vi "AlliGator FLI Dataset Actions.vi"(0 "AlliGator Q Elements":T6[](array[typedef]), 1 "VI in":refnum<vi>, 2 "Script in":bool, 5 "AlliGator IV DVR in":refnum<data-value>, 7 "AlliGator Q Event in":T7=enum."GUI:Idle", 9 "Data":variant, 11 "error in (no error)":errorcluster, 12 "AlliGator Ctrl Refnums":T8) -> (3 "Script out":bool, 4 "Alligator Queue Elements":T6[](array[typedef]), 6 "AlliGator IV DVR out":refnum<data-value>, 10 "[Notebook Message]":T1[](array[typedef]) {"Message Style"."Font Size" min=6.0 step=1.0}, 15 "error out":errorcluster)   [LabVIEW 2021, in "AlliGator Action Engine.lvlib"]
doc: "Processes AlliGator FLI Dataset-related actions."
uses:
  AlliGator Action Engine.lvlib
  Internal Variables/AlliGator Internal Variables v2.ctl
  <vilib>/vision/Image Controls.llb/IMAQ Image.ctl
  Internal Variables/AlliGator Gate Image Set.ctl
  Files/AlliGator FLI Dataset Type.ctl
  Files/AlliGator Data Series Type.ctl
  Dual-Channel Datasets/AlliGator Dataset Channel.ctl
  Settings/AlliGator Gate Arithmetic.ctl
  Source Image/AlliGator Displayed Image.ctl
  Image/Named ROI Description.ctl
  Phasor Graph/AlliGator Decay Metadata v3.ctl
  Decay Analysis/Decay Preprocessing/AlliGator Decay Background Subtraction Info.ctl
  Decay Analysis/Decay Preprocessing/AlliGator Baseline Subtraction Method.ctl
  Graphs/XY Graph/XY Graph Plot Shift Parameters.ctl
  Graphs/XY Graph/XY Graph Plot Shift Method.ctl
  Decay Analysis/Decay Preprocessing/AlliGator Decay Extrapolation Parameters.ctl
  Phasor/Calibration Phasor (m, phi).ctl
  Phasor/Phasor Reference Series.ctl
  Phasor/Phasor Calibration Map v2.ctl
  Phasor/Phasor (g, s).ctl
  Phasor Graph/AlliGator Raw Phasor Plot Data v5.ctl
  Phasor/Phasor Standard Deviation Options.ctl
  Phasor Plot/AlliGator Phasor Multi-Harmonic Data.ctl
  Phasor/Phasor Harmonic Data.ctl
  Decay Fit Parameter Map/AlliGator Decay Fit Options & Parameters v3.ctl
  Fits/IRF(X)PSED/Decay Fit Options v3.ctl
  Fits/Decay Convolution/Decay Model.ctl
  Fits/Residual Type.ctl
  Fits/IRF(X)PSED/Fit Weights Type.ctl
  Fits/Non-linear Fitting Method v2.ctl
  Fits/Fit Calculation Method.ctl
  Fits/Non-linear Fitting Algorithm.ctl
  Decay Analysis/Decay Fit/AlliGator Decay Fit Parameter Constraints 2.ctl
  Fits/IRF(X)PSED/Decay Fit Parameters In List.ctl
  Fits/IRF(X)PSED/MLE Baseline Offset Type.ctl
  Decay Analysis/Decay Preprocessing/AlliGator Decay Preprocessing Parameters.ctl
  Fits/IRF(X)PSED/Decay Fit Parameters & Derived Quantities List v2.ctl
  Fits/IRF(X)PSED/Decay Fit Result Constraint.ctl
  Decay Fit Parameter Map/AlliGator Parameter Maps Data.ctl
  AlliGator Q Event.ctl
  GUI/AlliGator Ctrl Refnums.ctl
  GUI/AlliGator Other Ctrl Refnums.ctl
  GUI/AlliGator State Indicator.ctl
  GUI/AlliGator Main Window Tabs.ctl
  GUI/AlliGator Phasor Plot Ctrl Refnums.ctl
  GUI/AlliGator Phasor Graph Ctrl Refnums.ctl
  Phasor/Phasor Calibration Type.ctl
  GUI/AlliGator Dataset Ctrl Refnums.ctl
  GUI/AlliGator Registered Events Ctrl Refnums.ctl
  GUI/AlliGator Image Histogram Control Refnums.ctl
  Histograms/Linear Histogram Options.ctl
  Histograms/Histogram Bin Option.ctl
  Histograms/Histogram Bin Position.ctl
  Decay Fit Parameter Map/AlliGator Decay Fit Map Control Refnums.ctl
  Parameter Map/AlliGator Parameter Map Control Refnums.ctl
  AlliGator Q Element.ctl
  Notebook/Notebook Message Object.ctl
  Rich Text Box/Text Formatting.ctl
  Rich Text Box/Text Colors.ctl
  Rich Text Box/Text Style.ctl
  Rich Text Box/Text Alignment.ctl
  AlliGator State Indicators List.ctl
  Alligator Elements Order in Action Stack.ctl
  Rich Text Box/Text Format List.ctl
  Graphs/Plot Point Style.ctl
  Graphs/LabVIEW Plot Interpolation.ctl
  Files/Load-Save File Info.ctl
  Dual-Channel Datasets/AlliGator Channel Arithmetic Action Parameters.ctl
  Scripts/AlliGator Multi-ROIs Dialog Type.ctl
  Image/Image Control ROI Description.ctl
  AlliGator Add Action Array to Stack.vi
  Variant/Variant to Data/Variant to Boolean.vi
  Graphs/XY Graph/XY Graph Add Single Plot with Name.vi
  Variant/Variant to Data/Variant to String.vi
  Image/Image.lvlib
  ROIs/AlliGator ROIs.lvlib
  Variant/Variant.lvlib
  Variant/Variant to Data/Variant to Data.lvlib
  GUI/GUI.lvlib
  Settings/AlliGator Settings.lvlib
  Dual-Channel Datasets/AlliGator Dual-Channel Datasets.lvlib
  Python Plugins API/AlliGator Python Plugins.lvlib
  Sound/Sound.lvlib
  Source Image/AlliGator Source Image.lvlib
  Scripts/AlliGator Scripts.lvlib
  Decay Analysis/IRF/AlliGator IRF.lvlib
  GUI/AlliGator GUI.lvlib
  Decay Analysis/Decay Fit/AlliGator Decay Fit.lvlib
  Decay Statistics/AlliGator Decay Statistics.lvlib
  Internal Variables/AlliGator Internal Variables.lvlib
  Decay Analysis/Decay Processing/AlliGator Decay Processing.lvlib
  Error/Error.lvlib
  Decay Fit Parameter Map/AlliGator Decay Fit Parameter Map.lvlib
  Phasor Graph/AlliGator Phasor Graph.lvlib
  Graphs/Graphs.lvlib
  Graphs/XY Graph/XY Graph Add-Ons.lvlib
  Files/Files.lvlib
  Notebook/Notebook.lvlib
  Phasor/Phasor.lvlib
  Decay Analysis/Decay Preprocessing/AlliGator Decay Preprocessing.lvlib
  Files/AlliGator Files.lvlib
  Phasor Plot/AlliGator Phasor Plot.lvlib
  Fits/Fits.lvlib
  Rich Text Box/Rich Text Box.lvlib
  Histograms/Histogram Window.lvlib
  Parameter Map/AlliGator Parameter Map.lvlib
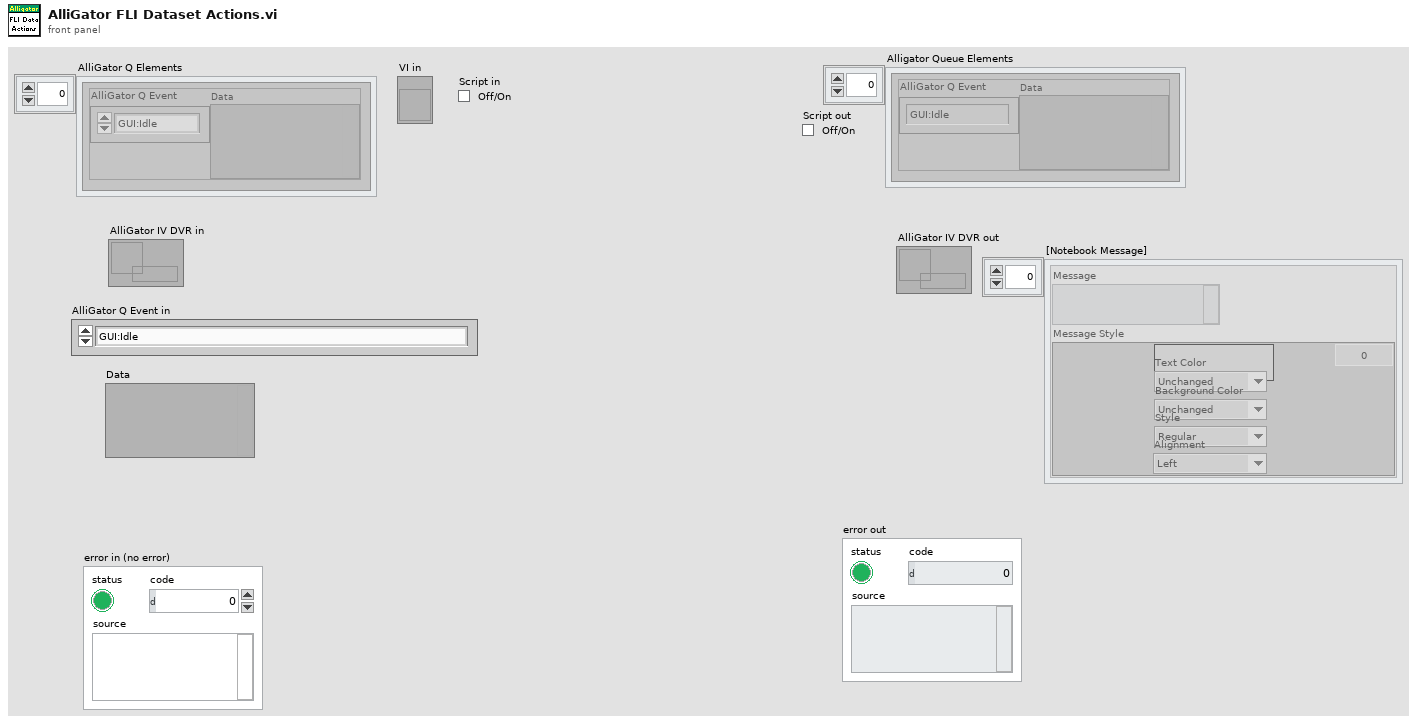
[diagram p1: front panel]
types:
  T1 = typedef "Notebook.lvlib/Notebook Message Object.ctl" = cluster{"Message":string, "Message Style":T2}
  T2 = typedef "Rich Text Box.lvlib/Text Formatting.ctl" = cluster{"Font":string, "Text Color":T3, "Background Color":T3, "Style":T4, "Font Size":dbl, "Alignment":T5}
  T3 = typedef "Rich Text Box.lvlib/Text Colors.ctl" = enum16{"Unchanged", "Black", "Blue", "Cyan", "Maroon", "Gray", "Violet", "Green", "Light Green", "Orange", "Yellow", "Magenta", "Red", "White"}
  T4 = typedef "Rich Text Box.lvlib/Text Style.ctl" = enum16{"Regular", "Bold", "Italic", "Underline", "Strikeout"}
  T5 = typedef "Rich Text Box.lvlib/Text Alignment.ctl" = enum16{"Left", "Right", "Center"}
  T6 = typedef "AlliGator Action Engine.lvlib/AlliGator Q Element.ctl" = cluster{"AlliGator Q Event":T7, "Data":variant}
  T7 = typedef "AlliGator Action Engine.lvlib/AlliGator Q Event.ctl" = enum16{"---- Files ----", "Files:Set Batch Export Files To Save", "Files:Set Dataset Loading & Pre-processing Options", "Files:Check #Frames in Dataset", "Files:Increment Frame Index", "Files:Open Mask Image", "Files:Open White Light Image", "Files:Open Single Dataset", "Files:New Folder of Folders Selected", "Files:Load File (all Types)_Scriptable", "Files:Move Flattened Series to Folders Series", "Files:Select Folder", "Files:Load FLI Dataset", "Files:Load Swiss SPAD 1 Dataset", "Files:Load Swiss SPAD 2 Dataset", "Files:Load .sdt FLI Dataset", "Files:Load .ptu FLI Dataset", "Files:Load .bin FLI Dataset", "Files:Load Single Gate Image Folder", "Files:Load I/m/phi Dataset (deprecated)", "Files:Load Single Image", "Files:Subtract Background File", "Files:Export FLI Dataset", "Files:Load HDF5 FLI Dataset", "Files:Set Destination File Path", "Files:Save Mask Image", "Files:Batch Conversion", "Files:New Folder Selected", "Files:Close FLI Dataset", "Files:Close FLI Dataset Series", "Files:Close White Light Image", "Files:Close Mask Image", "---- FLI Dataset ----", "FLI Dataset:Channel Arithmetic", "FLI Dataset:Export Average Lifetime Map as ASCII", "FLI Dataset:Export User-Defined Quantity Map as ASCII", "FLI Dataset:Python Function FLI Dataset Event", "FLI Dataset:ROI Analysis", "FLI Dataset:Tilted Logistic Square Gated IRF Characteristics Map", "FLI Dataset:Logistic Square Gated IRF Characteristics Map", "FLI Dataset:Square Gated IRF Characteristics Map", "FLI Dataset:Multi-ROI Single-Pixel Phasor Analysis", "FLI Dataset:Multi-ROI Single-Pixel NLSF Analysis", "FLI Dataset:All ROIs IRF Extraction", "FLI Dataset:All ROIs Decay Fit Non-Interactive (Fast + Individual IRF)", "FLI Dataset:All ROIs Phasor Analysis", "FLI Dataset:All ROIs Decay Fit", "FLI Dataset:Fluorescence Decay Statistics", "FLI Dataset:Update Decay Statistics Graph", "FLI Dataset:Get Decay from ROI", "FLI Dataset:All ROIs Average Lifetimes", "FLI Dataset:Save/Load Local IRFs", "FLI Dataset:Clear Local IRFs", "FLI Dataset:Phasor Calibration Maps (# Gates Series) Script", "FLI Dataset:Calibrated Phasor Map Series", "---- FLI Dataset Series ----", "FLI Dataset Series:Sum All Datasets in Series", "FLI Dataset Series:Add Dataset to Accumulated Dataset", "FLI Dataset Series:Display Accumulated Dataset", "FLI Dataset Series:Clear Dataset Series Sum", "FLI Dataset Series:Time-Series Analysis (NLSF)", "FLI Dataset Series:Time-Series Analysis (Phasor)", "---- Image ----", "Image:Update Image Profile Plots", "Image:Image Histogram Cursor Move", "Image:Image Histogram", "Image:Image Contrast", "Image:Set Image Histogram Cursor Move Flag", "Image:Clear Image Overlay", "Image:Use ROI as Search Area", "Image:Set ROI Diameter", "Image:Save Image Data as TIFF", "Image:Save Displayed Image with Overlay", "Image:Save Image Overlay Only", "Image:Save Image as Hot Pixel Mask", "Image:Change Source Image Color Palette", "Image:Copy Image to Clipboard", "Image:Source Image ROI Selection", "Image:Delete All ROIs", "Image:Delete All Unselected ROIs", "Image:Delete ROI", "Image:Merge All ROIs", "Image:Store ROI", "Image:Source Image ROI Storage", "Image:Export ROI Description to Notebook", "Image:Save ROI", "Image:Load ROI", "Image:Paste ROI Definition", "Image:Clear ROI", "Image:Identify ROIs in Mask Image", "Image:Create Complementary ROI", "Image:Create Contour ROI", "Image:Create ROI(s) from Pixels with Peak above Min_Scriptable", "Image:Create ROI(s) from Pixels with Intensity above Min_Scriptable", "Image:Compute ROI Statistics", "Image:Delete ROI(s) based on ROI Characteristics", "Image:Create ROI Grid", "Image:ROI to Individual Pixel ROIs", "Image:Python Function Source Image Event", "Image:Show Phasor Calibration Map ROI Centers", "Image:Convert ROI to Mask Image", "Image:Mouse Move", "Image:Mouse Up", "Image:Set Source Image Mouse Move Flag", "Image:Add Scale Bar Overlay", "Image:Delete Existing ROIs Option", "Image:Overlay ROI Median", "Image:Check Current ROI", "Image:Update True Pixel Value", "---- Decay ----", "Decay:Clear IRF/Reference Plot", "Decay:Add Decay to Graph", "Decay:Smoothen Plot", "Decay:Smoothen Plot Tail", "Decay:Average Selected Plots", "Decay:Extract IRF", "Decay:Optimal IRF Extraction", "Decay:Threshold IRF", "Decay:Fit to Model IRF", "Decay:Fit IRF to Square Gate", "Decay:Fit IRF to Logistic Square Gate", "Decay:Fit IRF to Tilted Logistic Square Gate", "Decay:Create Bounding Cursors Set", "Decay:Export Bounding Cursors Definition to Notebook", "Decay:Denoise Plot", "Decay:Compute Cumulative Function", "Decay:Use as Reference Decay", "Decay:Show Reference Decay/IRF", "Decay:Extrapolate Decay", "Decay:Create Head & Tail Bounding Cursors", "Decay:Store Cursor-defined Head & Tail Fractions", "Decay:Rebin Plot", "Decay:1-Normalize Decay", "Decay:[0-1]-Normalize Plot", "Decay:Straighten Decay", "Decay:Shift Decay", "Decay:Fold Decay", "Decay:Fit Decay", "Decay:Global Fit of Selected Decays", "Decay:Post Global Fit Script", "Decay:Add Global Fit Parameters to Graph", "Decay:Add Decay Parameter(s) to Plot (Graph)", "Decay:Export Decay to Phasor Graph", "Decay:Compute Average Lifetime", "Decay:Plot Convolution", "Decay:Graph Tip Strip Update", "---- Decay Statistics ----", "Decay Statistics:Tip Strip Update", "---- Intensity Time Trace ----", "Intensity Time Trace:Use File Timestamp", "Intensity Time Trace:Load Intensity Corrections File", "Intensity Time Trace:Clear Intensity Corrections File", "Intensity Time Trace:Tip Strip Update", "---- Phasor Plot ----", "Phasor Plot:Build Phasor Plot", "Phasor Plot:Change Phasor Plot Color Palette", "Phasor Plot:Adjust Phasor Plot Display Range", "Phasor Plot:Highlight Image ROI in Phasor Plot", "Phasor Plot:Save Phasor Plot Image with Overlay", "Phasor Plot:Export Complex Phasor Map", "Phasor Plot:Export Phasor Ratio Map", "Phasor Plot:Export Average Lifetime Map", "Phasor Plot:Compute Phase Lifetime Histogram", "Phasor Plot:Compute Phasor Ratio Histogram", "Phasor Plot:Compute Phase Lifetime vs Intensity Scatter Plot", "Phasor Plot:Weber 2-Component Decomposition", "Phasor Plot:Update Phasor Color Map Vertices", "Phasor Plot:Clear Phasor Overlay", "Phasor Plot:Use Segment Extremities as References", "Phasor Plot:Use UC/Segment Intersections as References", "Phasor Plot:Use UC/Principal Axis Intersections as References", "Phasor Plot:Use UC/Linear Fit Intersections as References", "Phasor Plot:Update Phasor Plot Reference", "Phasor Plot:Show Local Phasor Info in Phasor Plot", "Phasor Plot:Update Phasor Plot State", "Phasor Plot:Phasor Plot ROI Storage", "Phasor Plot:Phasor Plot ROI Selection", "Phasor Plot:Python Function Phasor Plot Event", "Phasor Plot:Overlay Phasor ROI, Ratio or Map in Source Image", "Phasor Plot:Compute Decay of Selected Phasors", "Phasor Plot:Phasor at Image Pixel", "Phasor Plot:Mouse Move", "Phasor Plot:Mouse Up", "Phasor Plot:Display Range Mouse Move", "Phasor Plot:Set Mouse Move Flag", "Phasor Plot:Update True Phasor Plot Value", "---- Phasor Graph ----", "Phasor Graph:Get Phasor Value", "Phasor Graph:Create New Phasor Plot Dialog", "Phasor Graph:Update Last Phasor Value", "Phasor Graph:Update Phasor (m, phi)", "Phasor Graph:Remove Single Phasor from Plot", "Phasor Graph:Add Single Phasor to Plot", "Phasor Graph:Remove Phasor Plot", "Phasor Graph:Remove Selected Phasor Plots", "Phasor Graph:Clear Phasor Data", "Phasor Graph:Clear Phasor Graph", "Phasor Graph:Cursor Move", "Phasor Graph:Draw Cursor Connecting Line", "Phasor Graph:Clear Cursor Connecting Line", "Phasor Graph:Find UC Intersection", "Phasor Graph:Use UC/Cursor-Defined Line Intersections", "Phasor Graph:Use Selected Plots Fitted Line/UC Intersections", "Phasor Graph:Use Selected Plots Principal Axis/UC Intersections", "Phasor Graph:Show Single Phasor", "Phasor Graph:Save Single Phasor Plot", "Phasor Graph:Save All Phasor Plots", "Phasor Graph:Load Phasor Plot(s)", "Phasor Graph:Phasor Multiplication", "Phasor Graph:Compute Average Phasor", "Phasor Graph:Compute Multiple Average Phasors (Selected Plots)", "Phasor Graph:Export Single Phasor Plot Phase Lifetimes", "Phasor Graph:Parameter 2 vs Parameter 1 Scatter Plot", "Phasor Graph:Use Cursor n Location", "Phasor Graph:Set Reference n to Current Phase Lifetime Value", "Phasor Graph:Set Reference n to Lifetime Value", "Phasor Graph:Set Cursor n Location", "Phasor Graph:Save Phasor Graph Image", "Phasor Graph:Update SEPL Plot", "Phasor Graph:Export Single Phasor Plot Data", "Phasor Graph:Export Selected Phasor Plots Data", "Phasor Graph:Python Function Phasor Graph Event", "Phasor Graph:Tip Strip Update", "---- Calibration ----", "Calibration:Set Calibration Type", "Calibration:Load/Save Phasor Calibration", "Calibration:Load/Save Phasor Calibration Series", "Calibration:Load/Save Phasor Calibration Map", "Calibration:Use as Calibration", "Calibration:Compute Optimal Calibration from Phasor References", "Calibration:Clear Phasor Calibration", "Calibration:Single Phasor Calibration Information", "Calibration:Use as Calibration Series", "Calibration:Use as Calibration Map", "Calibration:Clear Calibration Series", "Calibration:Phasor Calibration Series Information", "Calibration:Clear Calibration Map", "Calibration:Phasor Calibration Map Information", "Calibration:Apply Phasor Calibration", "Calibration:Update Single Plot Calibration", "Calibration:Update Multiple Plots Calibration", "Calibration:Clear Single Plot Calibration", "Calibration:Clear All Plots Calibrations", "Calibration:Clear Plot(s) Calibration(s)?", "---- Phasor Ratio ----", "Phasor Ratio:Clear Reference n", "Phasor Ratio:Toggle Selected Plot(s)  Lock to Reference 1", "Phasor Ratio:Use as Reference n", "Phasor Ratio:Send Reference n to Notebook", "Phasor Ratio:Toggle Selected Plot(s)  Lock to Reference 2", "Phasor Ratio:Compute Phasor Ratio at Mouse Location", "Phasor Ratio:Compute Phasor Plot's Average Phasor Ratio", "Phasor Ratio:Compute Time-Series Phasor Ratios", "Phasor Ratio:Fit Line to Phasor Ratio Plot", "Phasor Ratio:Save References", "Phasor Ratio:Load References", "Phasor Ratio:Update Phasor Reference 1", "Phasor Ratio:Update Phasor Reference 2", "Phasor Ratio:Move Cursor n to Reference n", "Phasor Ratio:Use as Phasor Reference 1 Lifetime", "Phasor Ratio:Use as Phasor Reference 2 Lifetime", "Phasor Ratio:Export Phasor Ratio Map as ASCII", "Phasor Ratio:Tip Strip Update", "---- Lifetime & Other Parameters Graph ----", "Lifetime:Compute Sliced Mean, SDV and CV Plots", "Lifetime:Plot Decay Shifts", "Lifetime:Plot Histogram", "---- Decay Fit Parameter Map ----", "Decay Fit Parameter Map:Export ROI NLSF Data as ASCII", "Decay Fit Parameter Map:Set Decay Fit Parameter Map Selection", "Decay Fit Parameter Map:Build Decay Fit Parameter Map", "Decay Fit Parameter Map:Change Decay Fit Parameter Map Color Palette", "Decay Fit Parameter Map:Export Decay Fit Parameter Map Data as ASCII", "Decay Fit Parameter Map:Export All Decay Fit Parameter Maps Data as ASCII", "Decay Fit Parameter Map:Selected Parameter Scatterplot", "Decay Fit Parameter Map:Parameter 2 vs Parameter 1 Scatterplot", "Decay Fit Parameter Map:Save Decay Fit Parameter Map Image", "Decay Fit Parameter Map:Save-Load IRFs & Fit Data", "Decay Fit Parameter Map:Update Local Decay Plots", "Decay Fit Parameter Map:Python Function Decay Fit Parameters Map Event", "Decay Fit Parameter Map:Overlay Decay Fit Parameter Map in Source Image", "Decay Fit Parameter Map:Selected Parameter vs Intensity Scatterplot", "Decay Fit Parameter Map:Mouse Up", "Decay Fit Parameter Map:Mouse Move", "Decay Fit Parameter Map:Display Range Mouse Move", "Decay Fit Parameter Map:Change Map Resolution", "Decay Fit Parameter Map:Variance Significance Maps", "Decay Fit Parameter Map:Fit Result Constraints Window", "---- Parameter Map ----", "Parameter Map:Export ROI Parameters Data as ASCII", "Parameter Map:Delete Parameter Map Set", "Parameter Map:Update Parameter List", "Parameter Map:Build Parameter Map", "Parameter Map:Change Parameter Map Color Palette", "Parameter Map:Export Parameter Map Data as ASCII", "Parameter Map:Export All Parameter Maps Data as ASCII", "Parameter Map:Selected Parameter Scatterplot", "Parameter Map:Parameter 2 vs Parameter 1 Scatterplot", "Parameter Map:Selected Parameter vs Intensity Scatterplot", "Parameter Map:Save Parameter Map Image", "Parameter Map:Save-Load IRFs & Parameter Maps (TODO)", "Parameter Map:Set Parameter Map Selection", "Parameter Map:Python Function Parameter Map Event", "Parameter Map:Overlay Parameter Map in Source Image", "Parameter Map:Update Local Decay Plots", "Parameter Map:Mouse Up", "Parameter Map:Mouse Move", "Parameter Map:Display Range Mouse Move", "---- Generic Graph ----", "Generic Graph:Generic XY Graph Event", "Generic Graph:Python Function XY Graph Event", "Generic Graph:New Plot", "Generic Graph:Save Plot", "Generic Graph:XY Plot Histogram", "Generic Graph:Set XY Graph Plot Name", "Generic Graph:Set Last Cursor Style", "Generic Graph:Tip Strip Update", "---- GUI ----", "GUI:Start Script", "GUI:Type of Displayed Image Changed", "GUI:Gate Image Slide Changed", "GUI:Show Busy Icon", "GUI:Show Busy Icon & Abort Button", "GUI:Hide Busy Icon", "GUI:Hide Busy Icon & Abort Button", "GUI:Abort", "GUI:End Script", "GUI:Start Timing", "GUI:End Timing", "GUI:Set State Indicator", "GUI:Send Parameters JSON Strings to Clipboard", "GUI:Set Gate Step", "GUI:Idle", "GUI:Initialization", "GUI:Quit", "GUI:Increment Dataset Index", "GUI:Set Dataset Index to -1", "GUI:Time Series Slider Moved", "GUI:Time Series Slider Changed", "GUI:Toggle Playback or Loop", "GUI:Playback Script", "GUI:Set Phasor Frequency", "GUI:Open Window", "GUI:Start Test Script", "GUI:End Test Script", "GUI:Set Verbose Mode", "GUI:Set Verbose Settings Mode", "DEBUG"}
  T8 = typedef "AlliGator GUI.lvlib/AlliGator Ctrl Refnums.ctl" = cluster{"Other AlliGator Ctrl Refnums":T9, "Phasor Plot Ctrl Refnums":T10, "Phasor Graph Ctrl Refnums":T11, "Dataset Control Refnums":T12, "Registered Events Ctrl Refnums":T13, "Image Histogram Ctrl Refnums":T14, "Decay Fit Map Ctrl Refnums":T15, "Parameter Map Ctrl Refnums":T16}
  T9 = typedef "AlliGator GUI.lvlib/AlliGator Other Ctrl Refnums.ctl" = cluster{"State Indicators":refnum<vi>, " Progress Bar":refnum<vi>, "Decay Graph Active":refnum<vi>, "Decay Statistics Bin":refnum<vi>, "Time Step":refnum<vi>, "Use File Timestamp":refnum<vi>, "Tab Control":refnum<vi>, "CPU":refnum<vi>, "Abort Fit":refnum<vi>, "Dataset File/Folder Path":refnum<vi>, "Abort ROI Creation":refnum<vi>, "Event LED":refnum<vi>, "Dataset File/Folder Path 2":refnum<vi>, "Dataset File/Folder Path 3":refnum<vi>, "Dataset File/Folder Path 4":refnum<vi>, "Dataset File/Folder Path 5":refnum<vi>, "Dataset File/Folder Path 6":refnum<vi>, "Dataset File/Folder Path 7":refnum<vi>, "Dataset File/Folder Path 8":refnum<vi>, "Dataset File/Folder Path 9":refnum<vi>, "Dataset File/Folder Path 10":refnum<vi>, "Dataset File/Folder Path 11":refnum<vi>}
  T10 = typedef "AlliGator GUI.lvlib/AlliGator Phasor Plot Ctrl Refnums.ctl" = cluster{"Phasor Ratio":refnum<vi>, "Modulus Lifetime":refnum<vi>, "Phasor at cursor (m, phi)":refnum<vi>, "Phase Lifetime":refnum<vi>, "Phasor at cursor (g, s)":refnum<vi>, "Phasor Plor Average Lifetime":refnum<vi>, "Phasor Plot Active":refnum<vi>, "Save Phasor Plot":refnum<vi>, "Image Overlay Color":refnum<vi>, "Phasor Plot Color Scale":refnum<vi>, "Reference 1 Button":refnum<vi>, "Reference 2 Button":refnum<vi>, "True Phasor Plot Value":refnum<vi>}
  T11 = typedef "AlliGator GUI.lvlib/AlliGator Phasor Graph Ctrl Refnums.ctl" = cluster{"Phasor Ratio":refnum<vi>, "Modulus Lifetime":refnum<vi>, "Phasor at cursor (m, phi)":refnum<vi>, "Phase Lifetime":refnum<vi>, "Phasor at cursor (g, s)":refnum<vi>, "Phasor Graph Average Lifetime":refnum<vi>, "Phasor Graph Active":refnum<vi>, "Save Phasor Graph":refnum<vi>, "Phasor Frame Slide":refnum<vi>, "Single Step Phasor":refnum<vi>, "Calibration Type":refnum<vi>, "Show Line":refnum<vi>, "Phase Lifetime 1":refnum<vi>, "Phase Lifetime 2":refnum<vi>, "Phasor Graph Frequency":refnum<vi>, "Phasor Reference 1 Control":refnum<vi>, "Phasor Reference 2 Control":refnum<vi>, "Calibration Lifetime":refnum<vi>, "Phase Lifetime SDV":refnum<vi>, "Average Lifetime SDV":refnum<vi>, "Phasor Ratio SDV":refnum<vi>, "Modulus Lifetime SDV":refnum<vi>}
  T12 = typedef "AlliGator GUI.lvlib/AlliGator Dataset Ctrl Refnums.ctl" = cluster{"Current Data":refnum<vi>, "Gate Image Slide":refnum<vi>, "Time Point Slide":refnum<vi>, "Current Time Stamp":refnum<vi>, "Save Image":refnum<vi>, "Displayed Image":refnum<vi>, "Overlay Mode":refnum<vi>, "Phasor Overlay Color":refnum<vi>, "Image Color Scale":refnum<vi>, "Use ROI as Search Area":refnum<vi>, "Source Image ROI Color":refnum<vi>, "True Pixel Value":refnum<vi>}
  T13 = typedef "AlliGator GUI.lvlib/AlliGator Registered Events Ctrl Refnums.ctl" = cluster{"Time Point Slider":refnum<vi>, "Phasor Plot Display Range":refnum<vi>, "Decay Graph":refnum<vi>, "Decay Statistics Graph":refnum<vi>, "Intensity Time Trace":refnum<vi>, "Phasor Graph":refnum<vi>, "Phasor Ratio Graph":refnum<vi>, "Lifetime Graph":refnum<vi>, "Phasor Plot Display":refnum<vi>, "Source Image Display":refnum<vi>, "Decay Fit Parameter Map Display Range":refnum<vi>, "Decay Fit Parameter Map Display":refnum<vi>, "Parameter Map Display Range":refnum<vi>, "Parameter Map Display":refnum<vi>, "Phasor Plot Display Range":refnum<vi>}
  T14 = typedef "AlliGator GUI.lvlib/AlliGator Image Histogram Control Refnums.ctl" = cluster{"Image Histogram":refnum<vi>, "Image Histogram Options":refnum<vi>, "Image Histogram Active":refnum<vi>, "Image Histogram Upper Percentile":refnum<vi>, "Image Histogram Lower Percentile":refnum<vi>, "Auto-Adjust Contrast":refnum<vi>}
  T15 = typedef "AlliGator Decay Fit Parameter Map.lvlib/AlliGator Decay Fit Map Control Refnums.ctl" = cluster{"Decay Fit Parameter Map Color Scale":refnum<vi>, "Decay Fit Parameter":refnum<vi>, "Max Parameter":refnum<vi>, "Min Parameter":refnum<vi>, "Decay Fit Parameter Map Display":refnum<vi>, "Decay Fit Parameter Map Display Range":refnum<vi>, "Decay Parameter Map X":refnum<vi>, "Decay Parameter Map Y":refnum<vi>, "Decay Parameter Map Value":refnum<vi>}
  T16 = typedef "AlliGator Parameter Map.lvlib/AlliGator Parameter Map Control Refnums.ctl" = cluster{"Parameter Map Color Scale":refnum<vi>, "Map Parameter":refnum<vi>, "Max Parameter":refnum<vi>, "Min Parameter":refnum<vi>, "Parameter Map Display":refnum<vi>, "Parameter Map Display Range":refnum<vi>, "Parameter Map Set":refnum<vi>, "Parameter Map X":refnum<vi>, "Parameter Map Y":refnum<vi>, "Parameter Map Value":refnum<vi>}
  T17 = typedef "Notebook.lvlib/Text Format List.ctl" = enum16{"Message", "Result", "Error", "Setting", "Verbose", "Warning"}
  T18 = typedef "AlliGator Action Engine.lvlib/Alligator Elements Order in Action Stack.ctl" = enum16{"Enqueue 2 AFTER 1", "Enqueue 2 BEFORE 1"}
  T19 = typedef "AlliGator Action Engine.lvlib/AlliGator State Indicators List.ctl" = enum16{"Phasor Calibration Defined", "Phasor Calibration Series Defined", "Phasor Calibration Map Defined", "Phasor Reference 1 Defined", "Phasor Reference 2 Defined", "Lifetime Reference 1 Defined", "Lifetime Reference 2 Defined", "Phasor Calibration Used", "Phasor Calibration Series Used", "Phasor Calibration Map Used", "Dataset Update Needed", "Phasor Plot Update Needed", "Reference/IRF Defined", "Individual IRFs Defined"}
  T20 = typedef "Graphs.lvlib/LabVIEW Plot Interpolation.ctl" = enum16{"Point (.)", "Stepwise Right (--.)", "Line + Point (\\. /)", "Stepwise Left (.--)", "Stepwise Centered (-.-)", "Stepwise Vertical (|.|)", "Line (-)", "Use Previous Plot's Style"}
  T21 = typedef "Graphs.lvlib/Plot Point Style.ctl" = enum16{"not defined", "None", "Empty Circle", "Filled Circle", "Thick Circle", "Dotted Circle", "Empty Square", "Filled Square", "Thick Square", "Dotted Square", "Small Filled Square", "Dot", "Cross", "Tiny Cross", "Large X", "Small x", "Diamond", "Small Empty Square"}
  T22 = typedef "Files.lvlib/Load-Save File Info.ctl" = cluster{"Load/Save":bool, "File Path":path}
  T23 = typedef "AlliGator Dual-Channel Datasets.lvlib/AlliGator Channel Arithmetic Action Parameters.ctl" = cluster{"Channel Name":u16, "Channel Arithmetic":T24}
  T24 = typedef "AlliGator Settings.lvlib/AlliGator Gate Arithmetic.ctl" = enum16{"None", "INT-G2", "G2/INT*<INT>", "(1 - G2/INT)*<INT>"}
  T25 = typedef "ROI Descriptor" = cluster{"Global Rectangle":i32[], "Contours":cluster{"ID":enum32{"External", "Internal"}, "Type":u32, "Coordinates":i32[]}[]}
  T26 = typedef "AlliGator Scripts.lvlib/AlliGator Multi-ROIs Dialog Type.ctl" = enum16{"Multi-ROIs Single-Pixel Phasor Analysis", "Multi-ROIs Single-Pixel NLSF Analysis", "Export ROI Fit Parameters as ASCII"}
  T27 = typedef "Image.lvlib/Image Control ROI Description.ctl" = cluster{"Image Control Label":string, "ROI Descriptor":T25}
  T28 = typedef "AlliGator GUI.lvlib/AlliGator State Indicator.ctl" = cluster{"Phasor Calibration Defined":bool, "Phasor Calibration Series Defined":bool, "Phasor Calibration Map Defined":bool, "Phasor Ratio Reference 1 Defined":bool, "Phasor Ratio Reference 2 Defined":bool, "Phasor Ratio Lifetime Reference 1 Defined ":bool, "Phasor Ratio Lifetime Reference 2 Defined":bool, "Phasor Calibration Used":bool, "Phasor Calibration Series Used":bool, "Phasor Calibration Map Used":bool, "Dataset Update Needed":bool, "Phasor Plot Update Needed":bool, "Reference/IRF Defined":bool, "Individual IRFs Defined":bool}
  T29 = typedef "IMAQ Image.ctl" = refnum<image>
  T30 = typedef "AlliGator Scripts.lvlib/AlliGator Data Load & Process Options.ctl" = cluster{"Data Information":T31, "Source Image Settings":T35, "Decay Preprocessing Options & Parameters":T42, "Clear Phasor Graph":bool}
  T31 = typedef "AlliGator Scripts.lvlib/AlliGator Data Information.ctl" = cluster{"Gates to Skip":T32, "# Gates":u32, "Gate Step":u32, "Gate Duration":dbl[unit], "Gate Separation":dbl[unit], "Pile-up Correction":bool, "Pixel Well Capacity":u32, "Define Gates to":T33, "Gates to Keep":T34, "Laser Period":dbl[unit], "SYNC Period":dbl[unit], "Channel Name":u16, "Channel Arithmetic":T24, "Background File Subtraction":bool, "Background Scaling Factor":dbl, "Background File":path, "Background Pile-up Correction":bool, "Background Pixel Well Capacity":u32, "Dataset Scaling Factor":dbl}
  T32 = typedef "AlliGator Settings.lvlib/AlliGator Background Subtraction Parameters.ctl" = cluster{"Start":u32, "End":u32}
  T33 = typedef "AlliGator Settings.lvlib/AlliGator Define Gates to.ctl" = enum32{"Skip", "Keep"}
  T34 = typedef "AlliGator Settings.lvlib/AlliGator Gates to Keep.ctl" = cluster{"First":u32, "Last":u32}
  T35 = typedef "AlliGator Scripts.lvlib/AlliGator Source Image Settings.ctl" = cluster{"Low Count Pixels Rejection Options":T36, "High Count Pixels Rejection Options":T37, "Peak Threshold":dbl, "Intensity Threshold":dbl, "Image Smoothing Options":T38, "Image Binning Options":T41}
  T36 = typedef "AlliGator Settings.lvlib/AlliGator Low Count Pixels Rejection Options.ctl" = cluster{"Background Low Threshold Factor":dbl, "Fixed Low Background Threshold":dbl, "Reject Low Count Pixels":bool, "Low Percentile":dbl}
  T37 = typedef "AlliGator Settings.lvlib/AlliGator High Count Pixels Rejection Options.ctl" = cluster{"Background High Threshold Factor":dbl, "Fixed High Background Threshold":dbl, "Reject High Count Pixels":bool, "High Percentile":dbl}
  T38 = typedef "AlliGator Settings.lvlib/AlliGator Image Smoothing Options.ctl" = cluster{"Use Image Smoothing":bool, "Kernel Type":T39, "Bin":i32, "Algorithm":T40}
  T39 = typedef "Arrays.lvlib/Kernel Type.ctl" = enum16{"Uniform", "Bilinear", "Gaussian"}
  T40 = typedef "Arrays.lvlib/Smoothing Algorithm.ctl" = enum16{"Rapid", "Thorough"}
  T41 = typedef "AlliGator Source Image.lvlib/AlliGator Image Binning Options.ctl" = cluster{"Use Image Binning":bool, "X Bin":i32, "Y Bin":i32}
  T42 = typedef "AlliGator Decay Preprocessing.lvlib/AlliGator Decay Preprocessing Options.ctl" = cluster{"Background Subtraction Parameters":T43, "Decay Preprocessing Parameters":T45, "Preprocessing Steps Order":string[]}
  T43 = typedef "AlliGator Decay Preprocessing.lvlib/AlliGator Background Subtraction Parameters.ctl" = cluster{"Background Definition Range":cluster{"Min Gate":dbl[unit], "Max Gate":dbl[unit]}, "Baseline Subtraction Method":T44, "Background Subtraction?":bool, "Background File":path, "Background Constant":dbl, "Background Scaling Factor":dbl, "Background Pile-up Correction":bool, "Background Pixel Well Capacity":u32}
  T44 = typedef "AlliGator Decay Preprocessing.lvlib/AlliGator Baseline Subtraction Method.ctl" = enum16{"Mean", "Min", "Square Gated Single-Exponential", "File", "Constant"}
  T45 = typedef "AlliGator Decay Preprocessing.lvlib/AlliGator Decay Preprocessing Parameters.ctl" = cluster{"Background Subtraction":bool, "Straighten Decay":bool, "Reverse Gates":bool, "1-Normalized Decay":bool, "Smoothen Decay":bool, "Smoothing Parameter":dbl, "Shift Decay":bool, "Decay Shift Parameters":T46, "Extrapolate Decay":bool, "Additional Points":u32, "Head Fraction":dbl, "Pixel-Normalize Decay":bool, "Use Periodicity":bool, "Use Cursors":bool, "Tail Fraction":dbl, "Use Decay Pre-Processing":bool, "Fold Decay":bool, "# Folds":u32, "[0-1]-Normalized Decay":bool}
  T46 = typedef "XY Graph Add-Ons.lvlib/XY Graph Plot Shift Parameters.ctl" = cluster{"Type":T47, "Shift":dbl[unit], "Threshold":dbl, "Rotate":bool}
  T47 = typedef "XY Graph Add-Ons.lvlib/XY Graph Plot Shift Method.ctl" = enum16{"Default", "CFD", "Threshold", "Cross-Correlation"}
  T48 = typedef "Fits.lvlib/Decay Fit Parameters & Derived Quantities List v2.ctl" = enum16{"Offset", "Baseline", "A_1", "tau_1", "A_2", "tau_2", "<tau>_a", "f1_a", "f2_a", "<tau>_i", "f1_i", "f2_i", "-", "R^2", "Chi^2"}
  T49 = typedef "AlliGator Phasor Graph.lvlib/AlliGator Phasor Plot Scatter Plot Parameters.ctl" = cluster{"Parameter 2":T50, "Parameter 1":T50}
  T50 = typedef "AlliGator Phasor Graph.lvlib/AlliGator Phasor Graph Parameter List.ctl" = enum16{"Time Stamp", "Index", "Phasor Parameters", "Phasor g", "Phasor s", "Phasor phi", "Phasor m", "Modulus Lifetime", "Phase Lifetime", "ROI Parameters", "ROI Center x", "ROI Center y", "ROI # pixels ", "Decay Parameters", "Intensity", "Background/Gate", "Intensity - Background", "Fitted Lifetime", "Fitted Intensity", "Phasor Ratio Parameters", "Amplitude Phasor Ratio", "Intensity Phasor Ratio", "Amplitude-Averaged Lifetime", "Intensity-Averaged Lifetime", "-", "Phasor Parameters SDV", "Phasor g SDV", "Phasor s SDV", "Phasor phi SDV", "Phasor m SDV", "Phase Lifetime SDV", "Modulus Lifetime SDV", "Phasor Ratio Parameters SDV", "Amplitude Phasor Ratio SDV", "Intensity Phasor Ratio SDV", "Amplitude-Averaged Lifetime SDV", "Intensity-Averaged Lifetime SDV"}
  T51 = typedef "AlliGator Scripts.lvlib/AlliGator Dataset + Calibration Map + Gate Step.ctl" = cluster{"Phasor Calibration Map Path":path, "Gate Step":i32, "Dataset Path":path}
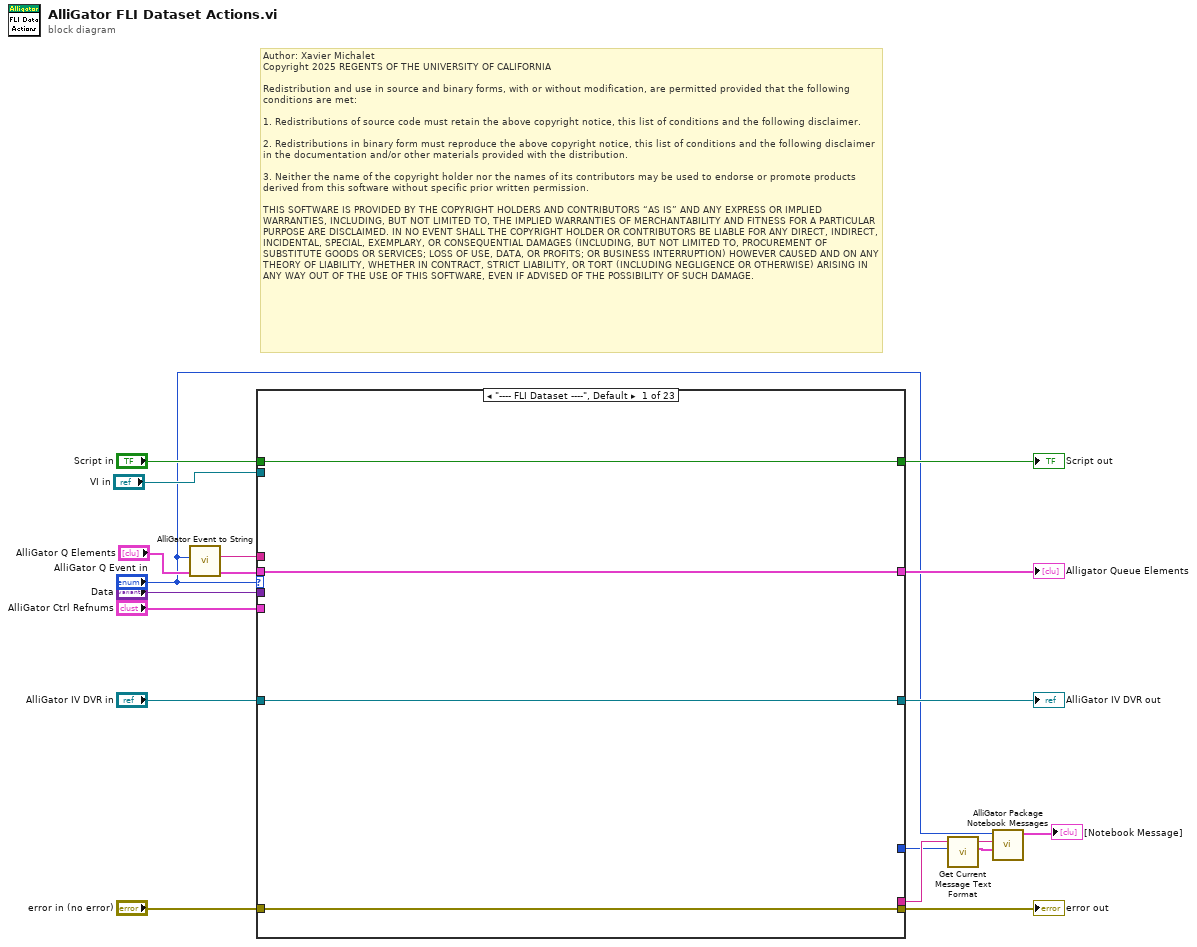
[diagram p0: block diagram]
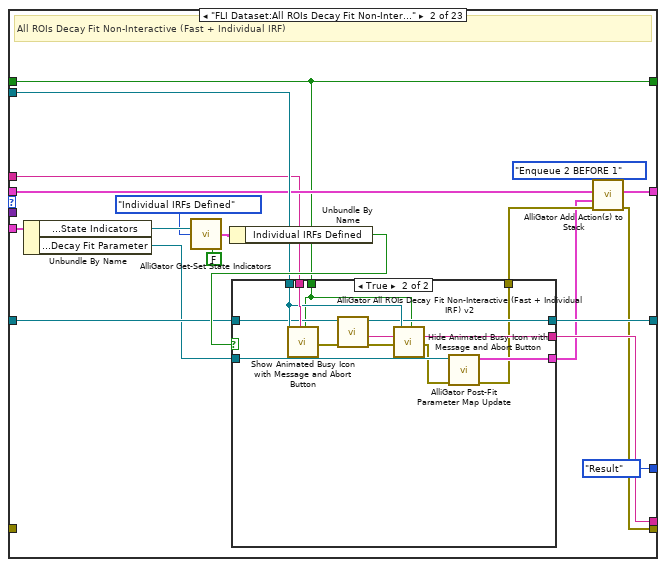
[diagram p2: hidden frame]
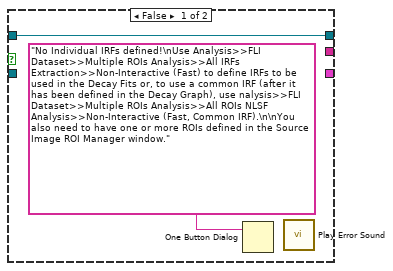
[diagram p3: hidden frame]
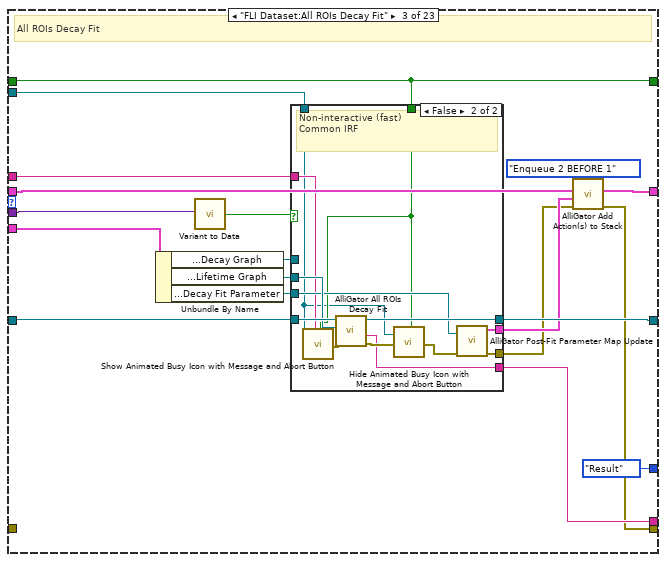
[diagram p4: hidden frame]
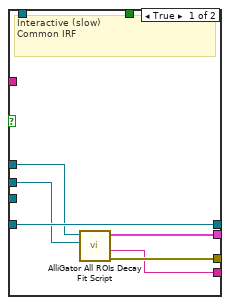
[diagram p5: hidden frame]
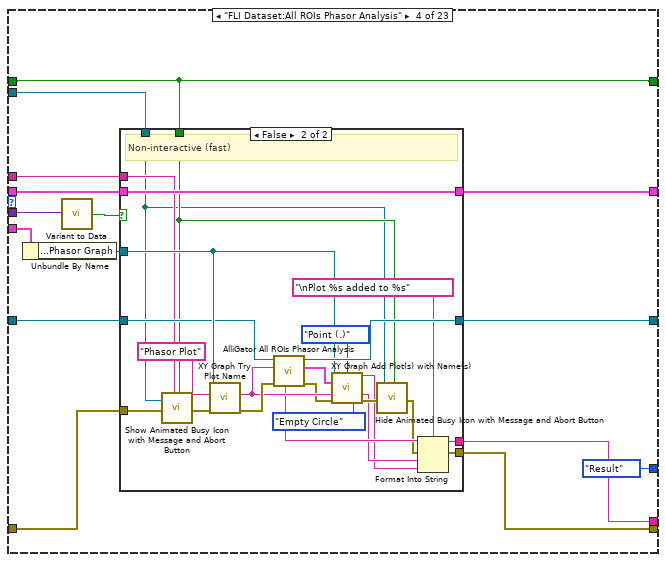
[diagram p6: hidden frame]
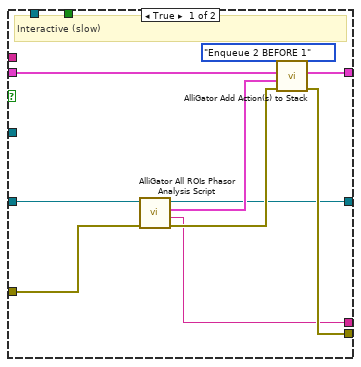
[diagram p7: hidden frame]
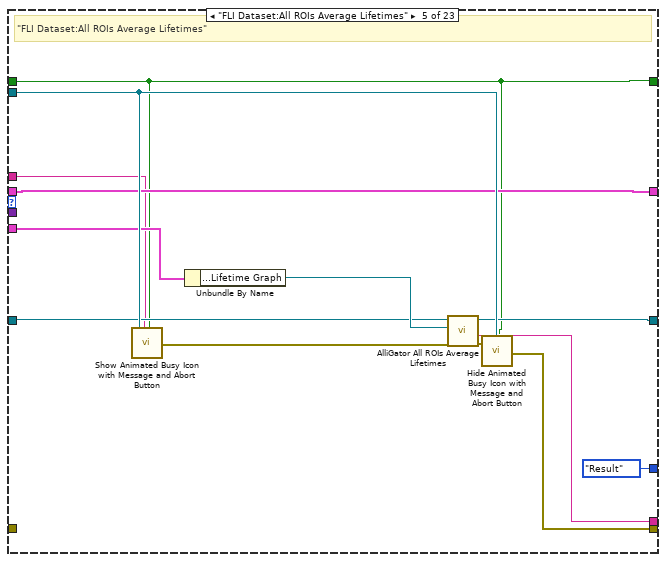
[diagram p8: hidden frame]
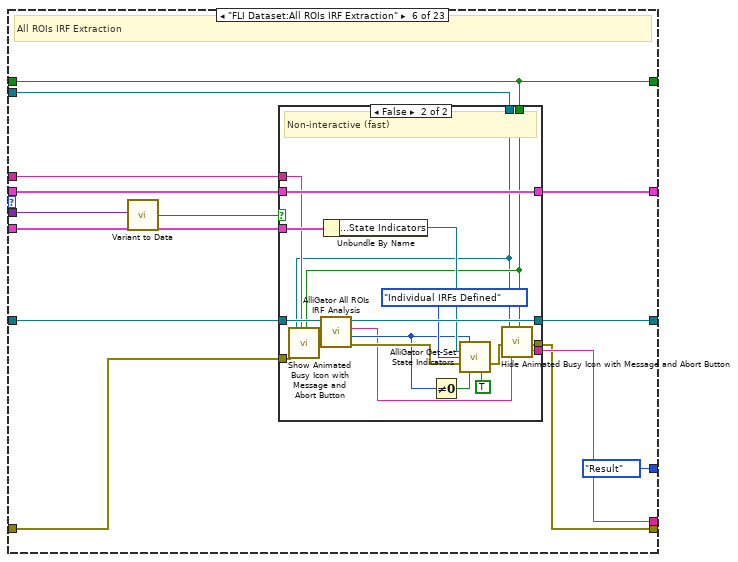
[diagram p9: hidden frame]
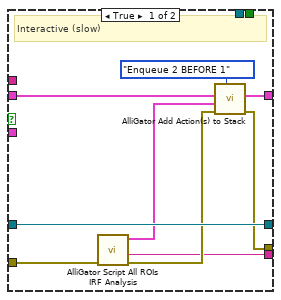
[diagram p10: hidden frame]
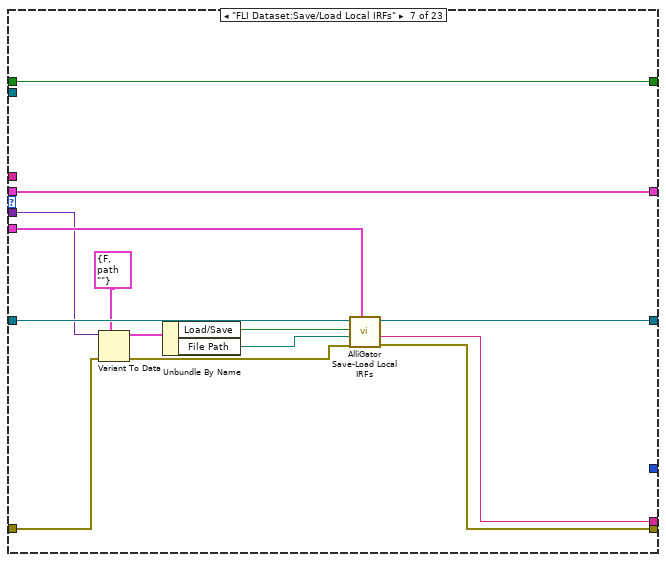
[diagram p11: hidden frame]
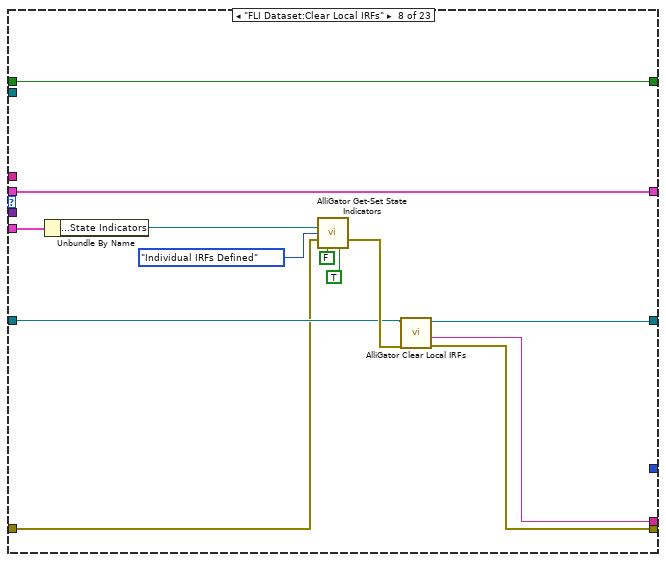
[diagram p12: hidden frame]
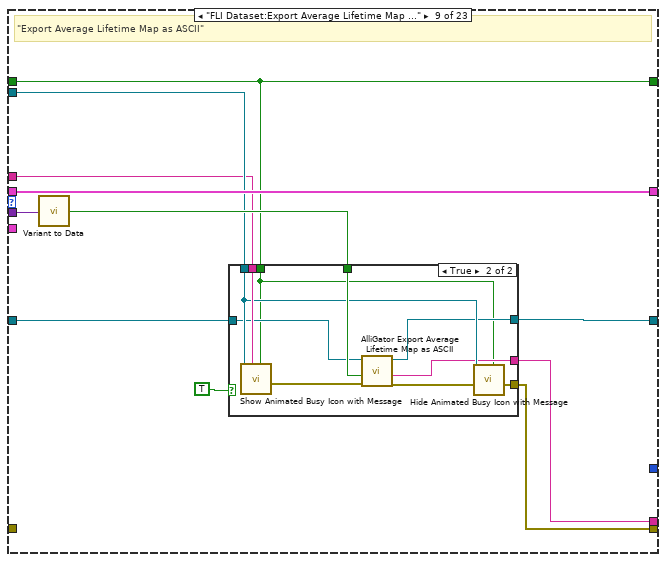
[diagram p13: hidden frame]
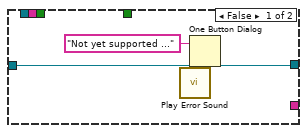
[diagram p14: hidden frame]
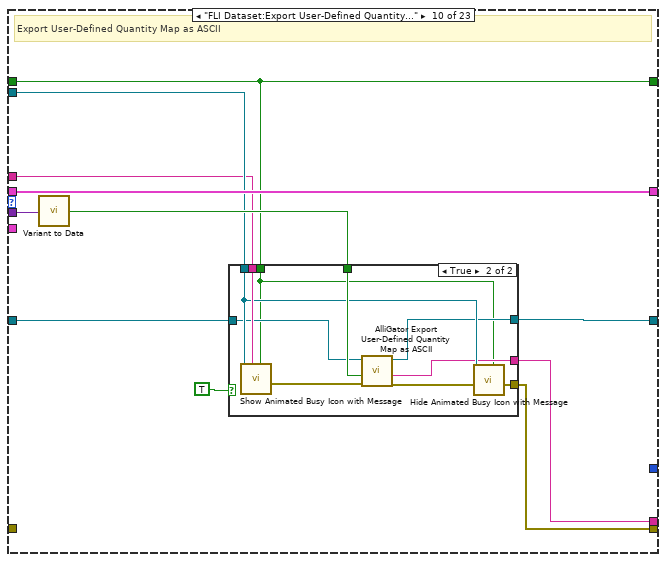
[diagram p15: hidden frame]
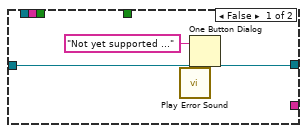
[diagram p16: hidden frame]
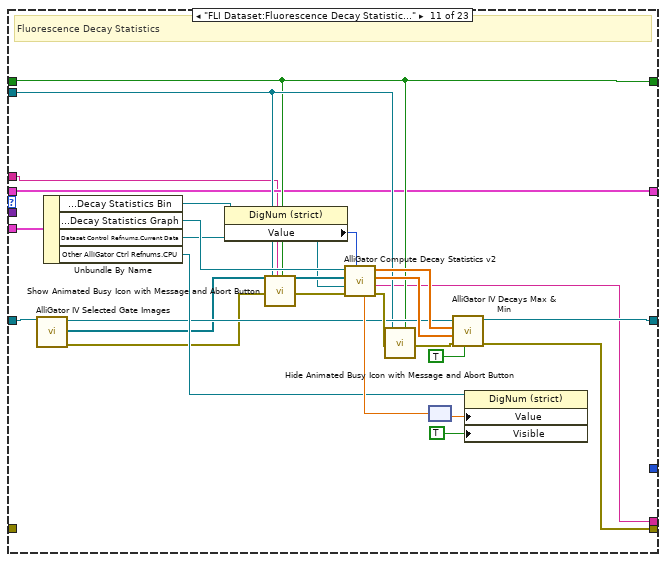
[diagram p17: hidden frame]
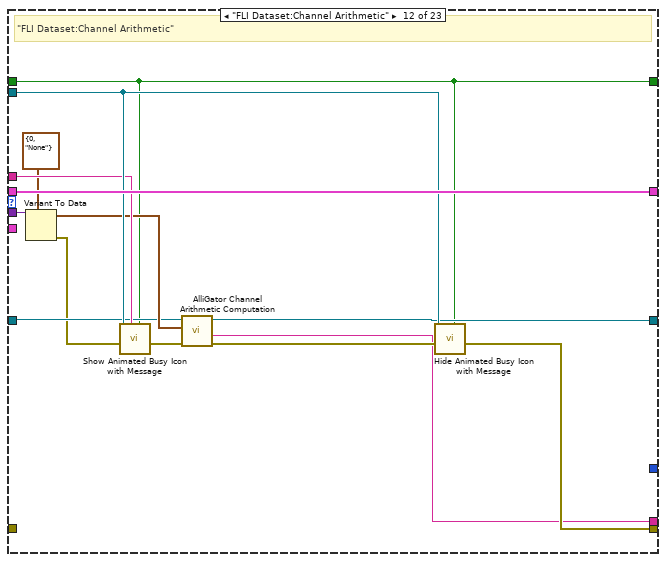
[diagram p18: hidden frame]
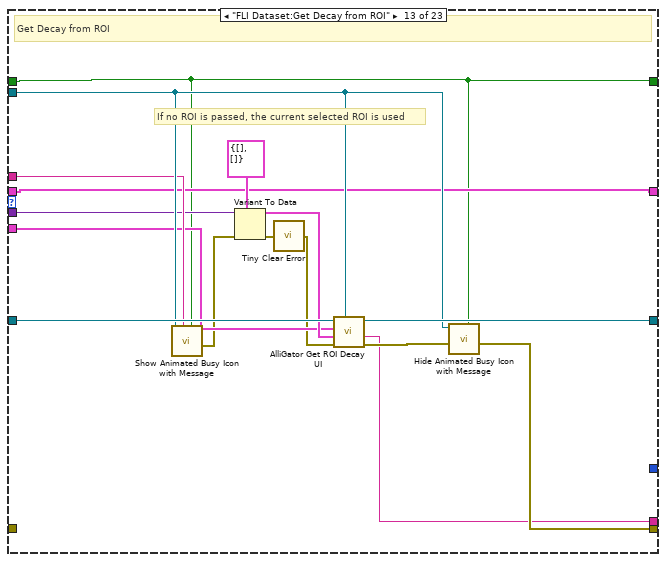
[diagram p19: hidden frame]
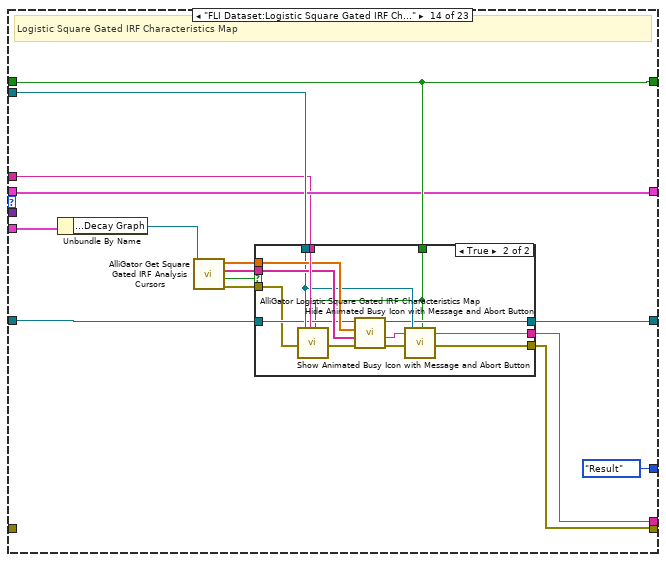
[diagram p20: hidden frame]
diagram:
  # "Author: Xavier Michalet\nCopyright 2025 REGENTS OF THE UNIVERSITY OF CALIFORNIA\n\nRedistribution and use in source and binary forms, with or without modification, are permitted provided that the following conditions are met:\n\n1. Redistributions of source code must retain the above copyright notice, this list of conditions and the following disclaimer.\n\n2. Redistributions in binary form must reproduce the above copyright notice, this list of conditions and the following disclaimer in the documentation and/or other materials provided with the distribution.\n\n3. Neither the name of the copyright holder nor the names of its contributors may be used to endorse or promote products derived from this software without specific prior written permission.\n\nTHIS SOFTWARE IS PROVIDED BY THE COPYRIGHT HOLDERS AND CONTRIBUTORS “AS IS” AND ANY EXPRESS OR IMPLIED WARRANTIES, INCLUDING, BUT NOT LIMITED TO, THE IMPLIED WARRANTIES OF MERCHANTABILITY AND FITNESS FOR A PARTICULAR PURPOSE ARE DISCLAIMED. IN NO EVENT SHALL THE COPYRIGHT HOLDER OR CONTRIBUTORS BE LIABLE FOR ANY DIRECT, INDIRECT, INCIDENTAL, SPECIAL, EXEMPLARY, OR CONSEQUENTIAL DAMAGES (INCLUDING, BUT NOT LIMITED TO, PROCUREMENT OF SUBSTITUTE GOODS OR SERVICES; LOSS OF USE, DATA, OR PROFITS; OR BUSINESS INTERRUPTION) HOWEVER CAUSED AND ON ANY THEORY OF LIABILITY, WHETHER IN CONTRACT, STRICT LIABILITY, OR TORT (INCLUDING NEGLIGENCE OR OTHERWISE) ARISING IN ANY WAY OUT OF THE USE OF THIS SOFTWARE, EVEN IF ADVISED OF THE POSSIBILITY OF SUCH DAMAGE."
  n1 = call "AlliGator Event to String.vi"("AlliGator Q Event"="AlliGator Q Event in") -> ("String"=w7:string)  [unwired: 8 in]
  n2 = case shown="\"---- FLI Dataset ----\", Default" "AlliGator Q Event in" {
    tunnel: "Data" -> [_ _ w70 w101 _ w166 w201 _ w233 w256 _ w306 w317 _ _ _ w470 _ _ _ _ _ _]
    tunnel: "AlliGator Q Elements" -> [w21 w35 w59 w106 w147 w167 w210 w223 w234 w257 w276 w309 w318 w333 w360 w436 w485 w511 w520 w530 w555 w577 w611]
    tunnel: [w21 w28 w65 w105 w147 w163 w210 w223 w234 w257 w276 w309 w318 w333 w362 w435 w484 w510 w520 w530 w555 w576 w607] -> w9
    tunnel: "VI in" -> [_ w36 w71 w100 w153 w168 _ _ w228 w251 w278 w308 w320 w335 _ _ w486 _ w519 w532 w559 w571 w605]
    tunnel: [w20 w23 w57 w95 w144 w157 w209 w222 w230 w253 w277 w296 w313 w334 w356 w437 w468 w504 w513 w531 w552 w570 w603] -> w10
    tunnel: "Script in" -> [w20 w23 w57 w95 w144 w157 w209 w222 w230 w253 w277 w296 w313 w334 w356 w437 w468 w504 w513 w531 w552 w570 w604]
    tunnel: w7 -> [_ w34 w58 w97 w146 w159 _ _ w224 w247 w275 w305 w319 w328 w359 _ w487 _ w518 w529 w553 w569 w602]
    tunnel: "error in (no error)" -> [w19 _ _ w96 _ w158 w203 w211 _ _ _ _ _ _ _ w431 _ _ _ _ _ w573 w608]
    tunnel: [w19 w25 w62 w99 w150 w160 w206 w213 w231 w254 w272 w304 w315 w329 w364 w433 w481 w503 w514 w526 w554 w574 w609] -> w6
    tunnel: "AlliGator Ctrl Refnums" -> [_ w33 w69 w98 w152 w165 w204 w216 _ _ w270 _ w316 w327 w361 w432 w475 w502 _ w528 w558 w572 w610]
    tunnel: "AlliGator IV DVR in" -> [w18 w32 w68 w104 w151 w164 w208 w215 w227 w250 w274 w301 w324 w332 w358 w450 w479 w489 w517 w527 w557 w585 w619]
    tunnel: [w18 w30 w66 w103 w148 w162 w207 w214 w226 w249 w273 w299 w325 w331 w357 w450 w478 w489 w516 w524 w556 w585 w619] -> w17
    tunnel: [_ w31 w67 w102 w149 w161 w205 w212 w225 w248 w271 w297 w314 w330 w363 w434 w476 _ w515 w525 _ w575 w606] -> w4
    tunnel: [_ Text_Format_List."Result" ("Text Format") Text_Format_List."Result" ("Text Format") Text_Format_List."Result" ("Text Format") Text_Format_List."Result" ("Text Format") Text_Format_List."Result" ("Text Format") _ _ _ _ _ _ _ Text_Format_List."Result" ("Text Format") Text_Format_List."Result" ("Text Format") Text_Format_List."Result" ("Text Format") Text_Format_List."Result" ("Text Format") Text_Format_List."Result" ("Text Format") Text_Format_List."Result" ("Text Format") Text_Format_List."Result" ("Text Format") _ _ _] -> w1
    frame "---- FLI Dataset ----", Default {
    }
    frame "FLI Dataset:All ROIs Decay Fit Non-Interactive (Fast + Individual IRF)" {
      # "All ROIs Decay Fit Non-Interactive (Fast + Individual IRF)"
      n3 = Unbundle By Name(w33) -> ("Other AlliGator Ctrl Refnums.State Indicators"=w41:refnum<vi>, "Decay Fit Map Ctrl Refnums.Decay Fit Parameter"=w29:refnum<vi>)
      n4 = call "AlliGator Get-Set State Indicators.vi"("State Indicators Refnum"=w41, "AlliGator State Indicators List"=AlliGator_State_Indicators_List."Individual IRFs Defined", "Set (T)/Get"=FALSE) -> ("State Indicator Values"=w38:T28)  [unwired: 10 in, 2 out]
      n5 = Unbundle By Name(w38) -> ("Individual IRFs Defined"=w37:bool)
      n6 = case shown="True" w37 {
        tunnel: w34 -> [_ w55]
        tunnel: w23 -> [_ w50]
        tunnel: [_ w44] -> w27
        tunnel: w36 -> [_ w53]
        tunnel: w32 -> [w42 w52]
        tunnel: [w42 w51] -> w30
        tunnel: [_ w49] -> w31
        tunnel: w29 -> [_ w48]
        tunnel: [_ w46] -> w26
        frame False {
          n7 = One Button Dialog(message="No Individual IRFs defined!\nUse Analysis>>FLI Dataset>>Multiple ROIs Analysis>>All IRFs Extraction>>Non-Interactive (Fast) to define IRFs to be used in the Decay Fits or, to use a common IRF (after it has been defined in the Decay Graph), use nalysis>>FLI Dataset>>Multiple ROIs Analysis>>All ROIs NLSF Analysis>>Non-Interactive (Fast, Common IRF).\n\nYou also need to have one or more ROIs defined in the Source Image ROI Manager window.") -> ()  [unwired: 1 in, 1 out]
          n8 = call "Play Error Sound.vi"() -> ()  [unwired: 27 in, 1 out]
        }
        frame True {
          n9 = call "Show Animated Busy Icon with Message and Abort Button.vi"("Already active? (F)"=w50, "Message"=w55, "Target VI reference"=w53) -> ("Error Out"=w54:errorcluster)  [unwired: 16 in]
          n10 = call "AlliGator All ROIs Decay Fit Non-Interactive (Fast + Individual IRF) v2.vi"("error in (no error)"=w54, "AlliGator Internal Variables DVR"=w52) -> ("error out"=w47:errorcluster, "Message"=w49:string, "AlliGator Internal Variables DVR"=w51:refnum<data-value>)  [unwired: 7 in]
          n11 = call "Hide Animated Busy Icon with Message and Abort Button.vi"("Already active? (F)"=w50, "Target VI reference"=w53, "Error In"=w47) -> ("Error Out"=w45:errorcluster)  [unwired: 16 in]
          n12 = call "AlliGator Post-Fit Parameter Map Update.vi"("Error In"=w45, "Decay Fit Parameter"=w48) -> ("Error Out"=w44:errorcluster, "Array of Actions"=w46:T6[])  [unwired: 8 in]
        }
      }
      n13 = call-poly "AlliGator Add Action(s) to Stack.vi"("Elements Order in Action Stack (Default: 2 BEFORE 1)"=Alligator_Elements_Order_in_Action_Stack."Enqueue 2 BEFORE 1", "Error In"=w27, "Alligator Queue Element 2"=w26, "Alligator Queue Element 1"=w35) -> ("Error Out"=w25:errorcluster, "Alligator Queue Element 1 (+ 2)"=w28:T6[])  [unwired: 6 in]
    }
    frame "FLI Dataset:All ROIs Decay Fit" {
      # "All ROIs Decay Fit"
      n14 = Unbundle By Name(w69) -> ("Registered Events Ctrl Refnums.Decay Graph"=w73:refnum<vi>, "Registered Events Ctrl Refnums.Lifetime Graph"=w72:refnum<vi>, "Decay Fit Map Ctrl Refnums.Decay Fit Parameter"=w61:refnum<vi>)
      n15 = call-poly "Variant to Data.vi"("Variant"=w70) -> ("Value"=w74:bool)  [unwired: 8 in]
      n16 = case shown="False" w74 {
        tunnel: w68 -> [w80 w93]
        tunnel: [w80 w92] -> w66
        tunnel: w71 -> [_ w82]
        tunnel: w57 -> [_ w84]
        tunnel: [w79 w87] -> w63
        tunnel: w73 -> [w78 _]
        tunnel: w72 -> [w77 w90]
        tunnel: [w76 w89] -> w67
        tunnel: [w75 w86] -> w64
        tunnel: w61 -> [_ w85]
        tunnel: w58 -> [_ w83]
        frame True {
          # "Interactive (slow)\nCommon IRF"
          n17 = call "AlliGator All ROIs Decay Fit Script.vi"("Lifetime Graph"=w77, "Decay Graph"=w78) -> ("Error Out"=w79:errorcluster, "Message"=w76:string, "All ROIs Decay Fit Script"=w75:T6[])  [unwired: 7 in]
        }
        frame False {
          # "Non-interactive (fast)\nCommon IRF"
          n18 = call "Show Animated Busy Icon with Message and Abort Button.vi"("Already active? (F)"=w84, "Message"=w83, "Target VI reference"=w82) -> ("Error Out"=w81:errorcluster)  [unwired: 16 in]
          n19 = call "AlliGator All ROIs Decay Fit.vi"("error in (no error)"=w81, "Lifetime Graph"=w90, "AlliGator Internal Variables DVR"=w93) -> ("error out"=w91:errorcluster, "Message"=w89:string, "AlliGator Internal Variables DVR"=w92:refnum<data-value>)  [unwired: 6 in]
          n20 = call "Hide Animated Busy Icon with Message and Abort Button.vi"("Already active? (F)"=w84, "Target VI reference"=w82, "Error In"=w91) -> ("Error Out"=w88:errorcluster)  [unwired: 16 in]
          n21 = call "AlliGator Post-Fit Parameter Map Update.vi"("Error In"=w88, "Decay Fit Parameter"=w85) -> ("Error Out"=w87:errorcluster, "Array of Actions"=w86:T6[])  [unwired: 8 in]
        }
      }
      n22 = call-poly "AlliGator Add Action(s) to Stack.vi"("Elements Order in Action Stack (Default: 2 BEFORE 1)"=Alligator_Elements_Order_in_Action_Stack."Enqueue 2 BEFORE 1", "Error In"=w63, "Alligator Queue Element 2"=w64, "Alligator Queue Element 1"=w59) -> ("Error Out"=w62:errorcluster, "Alligator Queue Element 1 (+ 2)"=w65:T6[])  [unwired: 6 in]
    }
    frame "FLI Dataset:All ROIs Phasor Analysis" {
      n23 = Unbundle By Name(w98) -> ("Registered Events Ctrl Refnums.Phasor Graph"=w107:refnum<vi>)
      n24 = call-poly "Variant to Data.vi"("Variant"=w101) -> ("Value"=w108:bool)  [unwired: 8 in]
      n25 = case shown="False" w108 {
        tunnel: w106 -> [w118 w130]
        tunnel: [w117 w130] -> w105
        tunnel: [w112 w142] -> w102
        tunnel: [w109 w141] -> w103
        tunnel: w96 -> [w116 w119]
        tunnel: w95 -> [_ w123]
        tunnel: [w114 w128] -> w99
        tunnel: w107 -> [_ w132]
        tunnel: w100 -> [_ w121]
        tunnel: w104 -> [w110 w125]
        tunnel: w97 -> [_ w122]
        frame True {
          # "Interactive (slow)"
          n26 = call "AlliGator All ROIs Phasor Analysis Script.vi"("Error In"=w116, "AlliGator Internal Variables DVR"=w110) -> ("Error Out"=w113:errorcluster, "All ROIs Analysis Message"=w112:string, "All ROIs Analysis Script"=w111:T6[], "AlliGator Internal Variables DVR"=w109:refnum<data-value>)  [unwired: 6 in]
          n27 = call-poly "AlliGator Add Action(s) to Stack.vi"("Elements Order in Action Stack (Default: 2 BEFORE 1)"=Alligator_Elements_Order_in_Action_Stack."Enqueue 2 BEFORE 1", "Error In"=w113, "Alligator Queue Element 2"=w111, "Alligator Queue Element 1"=w118) -> ("Error Out"=w114:errorcluster, "Alligator Queue Element 1 (+ 2)"=w117:T6[])  [unwired: 6 in]
        }
        frame False {
          # "Non-interactive (fast)"
          n28 = call "Show Animated Busy Icon with Message and Abort Button.vi"("Already active? (F)"=w123, "Message"=w122, "Target VI reference"=w121, "Error In"=w119) -> ("Error Out"=w120:errorcluster)  [unwired: 15 in]
          n29 = call "XY Graph Try Plot Name.vi"("Error In"=w120, "Plot Name in"="Phasor Plot", "XY Graph Refnum"=w132) -> ("Error Out"=w140:errorcluster, "Plot Name out"=w139:string)  [unwired: 5 in, 2 out]
          n30 = call "AlliGator All ROIs Phasor Analysis.vi"("error in (no error)"=w140, "New Plot Name"=w139, "AlliGator Internal Variables DVR"=w125) -> ("error out"=w131:errorcluster, "Phasor Plot"=w138:cluster{"g Array":dbl[], "s Array":dbl[]}, "AlliGator Internal Variables DVR"=w141:refnum<data-value>, "Message"=w137:string)  [unwired: 3 in, 2 out]
          n31 = call-poly "XY Graph Add Plot(s) with Name(s).vi"("XYGraph Ref in"=w132, "Plot Interpolation (Previous Plot's Style)"=LabVIEW_Plot_Interpolation."Point (.)", "Plot"=w138, "Plot Name (\"Plot\")"=w139, "error in (no error)"=w131, "Point Style (Dot)"=Plot_Point_Style."Empty Circle") -> ("XY Graph Caption (or Label)"=w133:string, "Plot Name"=w134:string, "error out"=w135:errorcluster)  [unwired: 6 in, 1 out]
          n32 = call "Hide Animated Busy Icon with Message and Abort Button.vi"("Already active? (F)"=w123, "Target VI reference"=w121, "Error In"=w135) -> ("Error Out"=w129:errorcluster)  [unwired: 16 in]
          n33 = Format Into String(format string="\nPlot %s added to %s", initial string=w137, error in=w129, w134, w133) -> (resulting string=w142:string, error out=w128:errorcluster)
        }
      }
    }
    frame "FLI Dataset:All ROIs Average Lifetimes" {
      # "\"FLI Dataset:All ROIs Average Lifetimes\""
      n34 = call "Show Animated Busy Icon with Message and Abort Button.vi"("Already active? (F)"=w144, "Message"=w146, "Target VI reference"=w153) -> ("Error Out"=w155:errorcluster)  [unwired: 16 in]
      n35 = Unbundle By Name(w152) -> ("Registered Events Ctrl Refnums.Lifetime Graph"=w154:refnum<vi>)
      n36 = call "AlliGator All ROIs Average Lifetimes.vi"("error in (no error)"=w155, "Lifetime Graph"=w154, "AlliGator Internal Variables DVR"=w151) -> ("error out"=w145:errorcluster, "Message"=w149:string, "AlliGator Internal Variables DVR"=w148:refnum<data-value>)  [unwired: 6 in]
      n37 = call "Hide Animated Busy Icon with Message and Abort Button.vi"("Already active? (F)"=w144, "Target VI reference"=w153, "Error In"=w145) -> ("Error Out"=w150:errorcluster)  [unwired: 16 in]
    }
    frame "FLI Dataset:All ROIs IRF Extraction" {
      # "All ROIs IRF Extraction"
      n38 = call-poly "Variant to Data.vi"("Variant"=w166) -> ("Value"=w169:bool)  [unwired: 8 in]
      n39 = case shown="False" w169 {
        tunnel: w167 -> [w178 w196]
        tunnel: [w177 w196] -> w163
        tunnel: w164 -> [w176 w195]
        tunnel: [w176 w194] -> w162
        tunnel: w158 -> [w175 w181]
        tunnel: w157 -> [_ w180]
        tunnel: [w173 w193] -> w160
        tunnel: w165 -> [_ w185]
        tunnel: w168 -> [_ w179]
        tunnel: [w170 w184] -> w161
        tunnel: w159 -> [_ w183]
        frame True {
          # "Interactive (slow)"
          n40 = call "AlliGator Script All ROIs IRF Analysis.vi"("Error In"=w175) -> ("Error Out"=w174:errorcluster, "Message"=w170:string, "All ROIs Analysis Script"=w172:T6[])  [unwired: 8 in]
          n41 = call-poly "AlliGator Add Action(s) to Stack.vi"("Elements Order in Action Stack (Default: 2 BEFORE 1)"=Alligator_Elements_Order_in_Action_Stack."Enqueue 2 BEFORE 1", "Error In"=w174, "Alligator Queue Element 2"=w172, "Alligator Queue Element 1"=w178) -> ("Error Out"=w173:errorcluster, "Alligator Queue Element 1 (+ 2)"=w177:T6[])  [unwired: 6 in]
        }
        frame False {
          # "Non-interactive (fast)"
          n42 = call "Show Animated Busy Icon with Message and Abort Button.vi"("Already active? (F)"=w180, "Message"=w183, "Target VI reference"=w179, "Error In"=w181) -> ("Error Out"=w182:errorcluster)  [unwired: 15 in]
          n43 = call "AlliGator All ROIs IRF Analysis.vi"("error in (no error)"=w182, "AlliGator Internal Variables DVR"=w195) -> ("error out"=w192:errorcluster, "# IRFs defined"=w188:i32, "Message"=w184:string, "AlliGator Internal Variables DVR"=w194:refnum<data-value>)  [unwired: 6 in]
          n44 = Unbundle By Name(w185) -> ("Other AlliGator Ctrl Refnums.State Indicators"=w190:refnum<vi>)
          n45 = Not Equal To 0?(x=w188) -> (x != 0?=w187:bool)
          n46 = call "AlliGator Get-Set State Indicators.vi"("# Defined IRFs"=w188, "State Indicators Refnum"=w190, "AlliGator State Indicators List"=AlliGator_State_Indicators_List."Individual IRFs Defined", "Error In"=w192, "ON/OFF"=w187, "Set (T)/Get"=TRUE) -> ("Error Out"=w191:errorcluster)  [unwired: 7 in, 2 out]
          n47 = call "Hide Animated Busy Icon with Message and Abort Button.vi"("Already active? (F)"=w180, "Target VI reference"=w179, "Error In"=w191) -> ("Error Out"=w193:errorcluster)  [unwired: 16 in]
        }
      }
    }
    frame "FLI Dataset:Save/Load Local IRFs" {
      n48 = Variant To Data(error in=w203, type=T22 {"Load/Save"=FALSE, "File Path"=path ""} ("Calibration File Information"), Variant=w201) -> (data=w199:T22, error out=w202:errorcluster)
      n49 = Unbundle By Name(w199) -> ("Load/Save"=w197:bool, "File Path"=w198:path)
      n50 = call "AlliGator Save-Load Local IRFs.vi"("AlliGator Ctrl Refnums"=w204, "error in (no error)"=w202, "File Path"=w198, "Save/Load (F)"=w197, "AlliGator IV DVR in"=w208) -> ("error out"=w206:errorcluster, "Message"=w205:string, "AlliGator IV DVR out"=w207:refnum<data-value>)  [unwired: 4 in]
    }
    frame "FLI Dataset:Clear Local IRFs" {
      n51 = Unbundle By Name(w216) -> ("Other AlliGator Ctrl Refnums.State Indicators"=w219:refnum<vi>)
      n52 = call "AlliGator Get-Set State Indicators.vi"("State Indicators Refnum"=w219, "AlliGator State Indicators List"=AlliGator_State_Indicators_List."Individual IRFs Defined", "Error In"=w211, "ON/OFF"=FALSE, "Set (T)/Get"=TRUE) -> ("Error Out"=w217:errorcluster)  [unwired: 8 in, 2 out]
      n53 = call "AlliGator Clear Local IRFs.vi"("error in (no error)"=w217, "AlliGator IV DVR in"=w215) -> ("error out"=w213:errorcluster, "Message"=w212:string, "AlliGator IV DVR out"=w214:refnum<data-value>)  [unwired: 7 in]
    }
    frame "FLI Dataset:Export Average Lifetime Map as ASCII" {
      # "\"Export Average Lifetime Map as ASCII\""
      n54 = call-poly "Variant to Data.vi"("Variant"=w233) -> ("Value"=w232:bool)  [unwired: 8 in]
      n55 = case shown="True" TRUE {
        tunnel: w232 -> [_ w246]
        tunnel: [_ w245] -> w231
        tunnel: w230 -> [_ w237]
        tunnel: w224 -> [_ w244]
        tunnel: w228 -> [_ w243]
        tunnel: w227 -> [w235 w242]
        tunnel: [w235 w240] -> w226
        tunnel: [_ w238] -> w225
        frame False {
          n56 = call "Play Error Sound.vi"() -> ()  [unwired: 27 in, 1 out]
          n57 = One Button Dialog(message="Not yet supported ...") -> ()  [unwired: 1 in, 1 out]
        }
        frame True {
          n58 = call "Show Animated Busy Icon with Message.vi"("Already active? (F)"=w237, "Message"=w244, "Target VI Refnum"=w243) -> ("Error Out"=w241:errorcluster)  [unwired: 8 in]
          n59 = call "AlliGator Export Average Lifetime Map as ASCII.vi"("error in (no error)"=w241, "Dialog?"=w246, "Data Value Reference in"=w242) -> ("error out"=w239:errorcluster, "Message"=w238:string, "Data Value Reference out"=w240:refnum<data-value>)  [unwired: 6 in]
          n60 = call "Hide Animated Busy Icon with Message.vi"("Already active? (F)"=w237, "Error In"=w239, "Target VI reference"=w243) -> ("Error Out"=w245:errorcluster)  [unwired: 8 in]
        }
      }
    }
    frame "FLI Dataset:Export User-Defined Quantity Map as ASCII" {
      # "Export User-Defined Quantity Map as ASCII"
      n61 = call-poly "Variant to Data.vi"("Variant"=w256) -> ("Value"=w255:bool)  [unwired: 8 in]
      n62 = case shown="True" TRUE {
        tunnel: w255 -> [_ w269]
        tunnel: [_ w268] -> w254
        tunnel: w253 -> [_ w260]
        tunnel: w247 -> [_ w267]
        tunnel: w251 -> [_ w266]
        tunnel: w250 -> [w258 w265]
        tunnel: [w258 w263] -> w249
        tunnel: [_ w261] -> w248
        frame False {
          n63 = call "Play Error Sound.vi"() -> ()  [unwired: 27 in, 1 out]
          n64 = One Button Dialog(message="Not yet supported ...") -> ()  [unwired: 1 in, 1 out]
        }
        frame True {
          n65 = call "Show Animated Busy Icon with Message.vi"("Already active? (F)"=w260, "Message"=w267, "Target VI Refnum"=w266) -> ("Error Out"=w264:errorcluster)  [unwired: 8 in]
          n66 = call "AlliGator Export User-Defined Quantity Map as ASCII.vi"("error in (no error)"=w264, "Dialog?"=w269, "Data Value Reference in"=w265) -> ("error out"=w262:errorcluster, "Message"=w261:string, "Data Value Reference out"=w263:refnum<data-value>)  [unwired: 6 in]
          n67 = call "Hide Animated Busy Icon with Message.vi"("Already active? (F)"=w260, "Error In"=w262, "Target VI reference"=w266) -> ("Error Out"=w268:errorcluster)  [unwired: 8 in]
        }
      }
    }
    frame "FLI Dataset:Fluorescence Decay Statistics" {
      # "Fluorescence Decay Statistics"
      n68 = call "AlliGator IV Selected Gate Images.vi"("AlliGator IV DVR in"=w274) -> ("Error Out"=w280:errorcluster, "Selected Gate Images"=w281:T29[], "AlliGator IV DVR out"=w282:refnum<data-value>)  [unwired: 8 in]
      n69 = Unbundle By Name(w270) -> ("Other AlliGator Ctrl Refnums.Decay Statistics Bin"=w292:refnum<vi>, "Registered Events Ctrl Refnums.Decay Statistics Graph"=w293:refnum<vi>, "Dataset Control Refnums.Current Data"=w279:refnum<vi>, "Other AlliGator Ctrl Refnums.CPU"=w290:refnum<vi>)
      n70 = property class="DigNum (strict)"(reference=w292) -> ("Value"=w291:i32)  [unwired: 1 in, 2 out]
      n71 = call "Show Animated Busy Icon with Message and Abort Button.vi"("Already active? (F)"=w277, "Message"=w275, "Target VI reference"=w278, "Error In"=w280) -> ("Error Out"=w295:errorcluster)  [unwired: 15 in]
      n72 = call "AlliGator Compute Decay Statistics v2.vi"("Decay Statistics Bin"=w291, "Error In"=w295, "Current Data"=w279, "Image Array"=w281, "Decay Statistics Graph Ref"=w293) -> ("Error Out"=w287:errorcluster, "Message"=w271:string, "Decays Min Values"=w285:sgl[], "Decays Max Values"=w286:sgl[], "Time (s)"=w294:dbl)  [unwired: 2 in]
      n73 = call "Hide Animated Busy Icon with Message and Abort Button.vi"("Already active? (F)"=w277, "Target VI reference"=w278, "Error In"=w287) -> ("Error Out"=w284:errorcluster)  [unwired: 16 in]
      n74 = node(w294) -> (w288:dbl[unit])
      n75 = call "AlliGator IV Decays Max & Min.vi"("Set (T)/Get (F)"=TRUE, "Error In"=w284, "[Decays Min Value]"=w285, "[Decays Max Value]"=w286, "AlliGator IV DVR in"=w282) -> ("Error Out"=w272:errorcluster, "AlliGator IV DVR out"=w273:refnum<data-value>)  [unwired: 3 in, 2 out]
      n76 = property class="DigNum (strict)"(reference=w290, "Value"=w288, "Visible"=TRUE) -> ()  [unwired: 1 in, 2 out]
    }
    frame "FLI Dataset:Channel Arithmetic" {
      # "\"FLI Dataset:Channel Arithmetic\""
      n77 = Variant To Data(type=T23 {"Channel Name"=0, "Channel Arithmetic"=enum."None"} ("Gate Arithmetic Action Parameters"), Variant=w306) -> (data=w302:T23, error out=w300:errorcluster)  [unwired: 1 in]
      n78 = call "Show Animated Busy Icon with Message.vi"("Already active? (F)"=w296, "Message"=w305, "Error In"=w300, "Target VI Refnum"=w308) -> ("Error Out"=w307:errorcluster)  [unwired: 7 in]
      n79 = call "AlliGator Channel Arithmetic Computation.vi"("Error In"=w307, "Channel Arithmetic Action Parameters"=w302, "AlliGator IV DVR in"=w301) -> ("Error Out"=w298:errorcluster, "Message"=w297:string, "AlliGator IV DVR out"=w299:refnum<data-value>)  [unwired: 6 in]
      n80 = call "Hide Animated Busy Icon with Message.vi"("Already active? (F)"=w296, "Error In"=w298, "Target VI reference"=w308) -> ("Error Out"=w304:errorcluster)  [unwired: 8 in]
    }
    frame "FLI Dataset:Get Decay from ROI" {
      # "If no ROI is passed, the current selected ROI is used"
      # "Get Decay from ROI"
      n81 = call "Show Animated Busy Icon with Message.vi"("Already active? (F)"=w313, "Message"=w319, "Target VI Refnum"=w320) -> ("Error Out"=w312:errorcluster)  [unwired: 8 in]
      n82 = Variant To Data(error in=w312, type=T25 {"Global Rectangle"=[], "Contours"=[]} ("ROI Descriptor"), Variant=w317) -> (data=w322:T25, error out=w311:errorcluster)
      n83 = call "Tiny Clear Error.vi"("Error In"=w311) -> ("no Error Out"=w310:errorcluster)  [unwired: 8 in]
      n84 = call "AlliGator Get ROI Decay UI.vi"("VI in"=w320, "error in (no error)"=w310, "ROI Descriptor"=w322, "AlliGator Ctrl Refnums"=w316, "AlliGator IV DVR"=w324) -> ("error out"=w321:errorcluster, "Message"=w314:string, "AlliGator IV DVR"=w325:refnum<data-value>)  [unwired: 4 in]
      n85 = call "Hide Animated Busy Icon with Message.vi"("Already active? (F)"=w313, "Error In"=w321, "Target VI reference"=w320) -> ("Error Out"=w315:errorcluster)  [unwired: 8 in]
    }
    frame "FLI Dataset:Logistic Square Gated IRF Characteristics Map" {
      # "Logistic Square Gated IRF Characteristics Map"
      n86 = Unbundle By Name(w327) -> ("Registered Events Ctrl Refnums.Decay Graph"=w336:refnum<vi>)
      n87 = call "AlliGator Get Square Gated IRF Analysis Cursors.vi"("XYGraph in"=w336) -> ("Error Out"=w340:errorcluster, "5 Cursors available?"=w337:bool, "Cursor Names Array"=w338:string[], "Cursor Positions Array"=w339:dbl[])  [unwired: 7 in]
      n88 = case shown="True" w337 {
        tunnel: w334 -> [_ w343]
        tunnel: w328 -> [_ w352]
        tunnel: w340 -> [w342 w346]
        tunnel: w339 -> [_ w351]
        tunnel: w338 -> [_ w350]
        tunnel: [w342 w345] -> w329
        tunnel: w335 -> [_ w349]
        tunnel: w332 -> [w341 w348]
        tunnel: [w341 w347] -> w331
        tunnel: [_ w344] -> w330
        frame False {
        }
        frame True {
          n89 = call "Show Animated Busy Icon with Message and Abort Button.vi"("Already active? (F)"=w343, "Message"=w352, "Target VI reference"=w349, "Error In"=w346) -> ("Error Out"=w354:errorcluster)  [unwired: 15 in]
          n90 = call "AlliGator Logistic Square Gated IRF Characteristics Map.vi"("error in (no error)"=w354, "Cursor Names Array"=w350, "Cursor Positions Array"=w351, "AlliGator Internal Variables DVR"=w348) -> ("error out"=w353:errorcluster, "Message"=w344:string, "AlliGator Internal Variables DVR"=w347:refnum<data-value>)  [unwired: 5 in]
          n91 = call "Hide Animated Busy Icon with Message and Abort Button.vi"("Already active? (F)"=w343, "Target VI reference"=w349, "Error In"=w353) -> ("Error Out"=w345:errorcluster)  [unwired: 16 in]
        }
      }
    }
    frame "FLI Dataset:Multi-ROI Single-Pixel NLSF Analysis" {
      # "Multi-ROI Single-Pixel NLSF Analysis"
      n92 = call "AlliGator NLSF & Phasor Multi-ROI Analysis Dialog.vi"("Dialog Type"=AlliGator_Multi-ROIs_Dialog_Type."Multi-ROIs Single-Pixel NLSF Analysis") -> ("Dataset Loading & Pre-processing Options"=w365:T30, "IRF Loading & Pre-processing Options"=w367:T30, "OK"=w370:bool, "IRF File"=w374:path, "Dataset File"=w373:path, "ROI File"=w372:path, "Decay Fit Parameters to Save"=w371:T48[], "Bins Array"=w368:dbl[], "Results Folder"=w376:path, "error out"=w377:errorcluster)  [unwired: 4 in, 1 out]
      n93 = Unbundle By Name(w361) -> ("Registered Events Ctrl Refnums.Lifetime Graph"=w369:refnum<vi>, "Registered Events Ctrl Refnums.Phasor Graph"=w375:refnum<vi>)
      n94 = case shown="True" w370 {
        tunnel: w360 -> [w380 w400]
        tunnel: [w380 w399] -> w362
        tunnel: w377 -> [w379 w384]
        tunnel: w375 -> [_ w398]
        tunnel: w359 -> [_ w402]
        tunnel: [w379 w401] -> w364
        tunnel: w374 -> [_ w387]
        tunnel: w373 -> [_ w397]
        tunnel: w372 -> [_ w396]
        tunnel: w371 -> [_ w395]
        tunnel: w376 -> [_ w394]
        tunnel: w369 -> [_ w393]
        tunnel: w368 -> [_ w392]
        tunnel: w367 -> [_ w391]
        tunnel: w365 -> [_ w390]
        tunnel: [_ w389] -> w363
        tunnel: w358 -> [w378 w388]
        tunnel: [w378 w383] -> w357
        frame False {
        }
        frame True {
          n95 = Empty String/Path?(string/path=w387) -> (empty?=w386:bool)
          n96 = case shown="True" w386 {
            tunnel: w388 -> [w423 w429]
            tunnel: w384 -> [w422 w428]
            tunnel: [w422 w427] -> w385
            tunnel: [w423 w426] -> w383
            tunnel: [_ w425] -> w381
            tunnel: [TRUE ("Valid Reference?") w424] -> w382
            frame False {
              # "indiv. IRFs"
            }
            frame True {
              # "single IRF"
              n97 = call "AlliGator Check Decay Reference.vi"("Error In"=w428, "AlliGator Internal Variables DVR"=w429) -> ("Error Out"=w427:errorcluster, "Valid Reference?"=w424:bool, "AlliGator Internal Variables DVR"=w426:refnum<data-value>, "Message"=w425:string)  [unwired: 2 in, 4 out]
            }
          }
          n98 = case shown="True" w382 {
            tunnel: w402 -> [_ _]
            tunnel: [w403 w417] -> w401
            tunnel: w400 -> [w404 w420]
            tunnel: [w404 w419] -> w399
            tunnel: w398 -> [_ w418]
            tunnel: w397 -> [_ w416]
            tunnel: w396 -> [_ w415]
            tunnel: w395 -> [_ w414]
            tunnel: w394 -> [_ w413]
            tunnel: w393 -> [_ w412]
            tunnel: w392 -> [_ w411]
            tunnel: w391 -> [_ w410]
            tunnel: w390 -> [_ w409]
            tunnel: [w405 w408] -> w389
            tunnel: w387 -> [_ w407]
            tunnel: w385 -> [w403 w406]
            tunnel: w381 -> [w405 _]
            frame False {
            }
            frame True {
              # "Valid IRF"
              n99 = call "AlliGator Script Multi-ROI Single-Pixel NLSF Analysis.vi"("Alligator Queue Elements in"=w420, "IRF File"=w407, "Dataset File"=w416, "ROI File"=w415, "Decay Fit Parameter to Save"=w414, "Error In"=w406, "Phasor Graph refnum"=w418, "Results Folder"=w413, "Lifetime Graph Refnum"=w412, "Bins Array"=w411, "IRF Loading & Pre-processing Options"=w410, "Dataset Loading & Pre-processing Options"=w409) -> ("Alligator Queue Elements out"=w419:T6[], "Message"=w408:string, "Error Out"=w417:errorcluster)  [unwired: 5 in]
            }
          }
        }
      }
    }
    frame "FLI Dataset:Multi-ROI Single-Pixel Phasor Analysis" {
      # "\"FLI Dataset:Multi-ROI Single-Pixel Phasor Analysis\""
      n100 = Unbundle By Name(w432) -> ("Registered Events Ctrl Refnums.Lifetime Graph"=w442:refnum<vi>, "Registered Events Ctrl Refnums.Phasor Graph"=w447:refnum<vi>)
      n101 = call "AlliGator NLSF & Phasor Multi-ROI Analysis Dialog.vi"("Dialog Type"=AlliGator_Multi-ROIs_Dialog_Type."Multi-ROIs Single-Pixel Phasor Analysis", "error in (no error)"=w431) -> ("Dataset Loading & Pre-processing Options"=w439:T30, "IRF Loading & Pre-processing Options"=w441:T30, "OK"=w443:bool, "IRF File"=w446:path, "Dataset File"=w445:path, "ROI File"=w444:path, "Phasor Parameters Scatter Plots"=w438:T49[], "Results Folder"=w448:path, "error out"=w449:errorcluster)  [unwired: 3 in, 2 out]
      n102 = case shown="True" w443 {
        tunnel: w436 -> [w452 w466]
        tunnel: [w452 w465] -> w435
        tunnel: w449 -> [w451 w462]
        tunnel: w447 -> [_ w464]
        tunnel: [w451 w463] -> w433
        tunnel: w446 -> [_ w461]
        tunnel: w445 -> [_ w460]
        tunnel: w444 -> [_ w459]
        tunnel: w448 -> [_ w458]
        tunnel: w442 -> [_ w457]
        tunnel: w441 -> [_ w456]
        tunnel: w439 -> [_ w455]
        tunnel: w438 -> [_ w454]
        tunnel: [_ w453] -> w434
        frame False {
        }
        frame True {
          n103 = call "AlliGator Script Multi-ROI Single-Pixel Phasor Analysis.vi"("Alligator Queue Elements in"=w466, "IRF File"=w461, "Dataset File"=w460, "ROI File"=w459, "Error In"=w462, "Phasor Graph refnum"=w464, "Results Folder"=w458, "Lifetime Graph Refnum"=w457, "IRF Loading & Pre-processing Options"=w456, "Phasor Parameters Scatter Plot"=w454, "Dataset Loading & Pre-processing Options"=w455) -> ("Alligator Queue Elements out"=w465:T6[], "Message"=w453:string, "Error Out"=w463:errorcluster)  [unwired: 6 in]
        }
      }
    }
    frame "FLI Dataset:Python Function FLI Dataset Event" {
      # "\"Python Function FLI Dataset Event\""
      n104 = Unbundle By Name(w475) -> ("Dataset Control Refnums.Current Data"=w474:refnum<vi>)
      n105 = call-poly "Variant to Data.vi"("Variant"=w470) -> ("String"=w469:string)  [unwired: 8 in]
      n106 = call "Show Animated Busy Icon with Message.vi"("Already active? (F)"=w468, "Message"=w487, "Target VI Refnum"=w486) -> ("Error Out"=w473:errorcluster)  [unwired: 8 in]
      n107 = property class="Str"(reference=w474, error in=w473) -> (error out=w472:errorcluster, "Value"=w471:string)  [unwired: 1 out]
      n108 = call "AlliGator FLI Dataset Python Function Handler Core.vi"("error in (no error)"=w472, "Current Data"=w471, "Data Value Reference in"=w479, "Item Tag"=w469) -> ("error out"=w477:errorcluster, "Message"=w476:string, "Data Value Reference out"=w478:refnum<data-value>, "Alligator Atomic Action"=w480:T6[])  [unwired: 4 in]
      n109 = call "Hide Animated Busy Icon with Message.vi"("Already active? (F)"=w468, "Error In"=w477, "Target VI reference"=w486) -> ("Error Out"=w483:errorcluster)  [unwired: 8 in]
      n110 = call-poly "AlliGator Add Action(s) to Stack.vi"("Elements Order in Action Stack (Default: 2 BEFORE 1)"=Alligator_Elements_Order_in_Action_Stack."Enqueue 2 BEFORE 1", "Error In"=w483, "Alligator Queue Element 2"=w480, "Alligator Queue Element 1"=w485) -> ("Error Out"=w481:errorcluster, "Alligator Queue Element 1 (+ 2)"=w484:T6[])  [unwired: 6 in]
    }
    frame "FLI Dataset:ROI Analysis" {
      # "\"ROI Analysis\""
      n111 = Unbundle By Name(w502) -> ("Phasor Graph Ctrl Refnums.Phasor Graph Active"=w493:refnum<vi>, "Other AlliGator Ctrl Refnums.Decay Graph Active"=w491:refnum<vi>, "Registered Events Ctrl Refnums.Source Image Display"=w501:refnum<vi>)
      n112 = call "Image Display Get-Set ROI.vi"("Get(F)/Set"=FALSE ("Get(F)/Set(T)"), "Image Display Refnum"=w501) -> ("Error Out"=w498:errorcluster, "Label.Text"=w497:string, "ROI Descriptor out"=w500:T25)  [unwired: 5 in, 2 out]
      n113 = call "Ctrl Refnum to Value (Variant).vi"("Ctl Refnum"=w493) -> ("Value"=w492:variant)  [unwired: 13 in, 1 out]
      n114 = call "Ctrl Refnum to Value (Variant).vi"("Ctl Refnum"=w491) -> ("Value"=w490:variant)  [unwired: 13 in, 1 out]
      n115 = call-poly "Variant to Data.vi"("Variant"=w492) -> ("Value"=w496:bool)  [unwired: 8 in]
      n116 = call-poly "Variant to Data.vi"("Variant"=w490) -> ("Value"=w495:bool)  [unwired: 8 in]
      n117 = Bundle By Name(cluster=T27 {"Image Control Label"="", "ROI Descriptor"={"Global Rectangle"=[], "Contours"=[]}}, "ROI Descriptor"=w500, "Image Control Label"=w497) -> (w506:T27)
      n118 = Compound Arithmetic op=OR(w496, w495) -> (w494:bool)
      n119 = call "AlliGator ROI Analysis Script.vi"("Error In"=w498, "Decay Graph OR Phasor Graph Active?"=w494, "Image ROI"=w506) -> ("Error Out"=w505:errorcluster, "ROI Analysis Script"=w508:T6[])  [unwired: 7 in]
      n120 = call-poly "AlliGator Add Action(s) to Stack.vi"("Elements Order in Action Stack (Default: 2 BEFORE 1)"=Alligator_Elements_Order_in_Action_Stack."Enqueue 2 BEFORE 1", "Error In"=w505, "Alligator Queue Element 2"=w508, "Alligator Queue Element 1"=w511) -> ("Error Out"=w503:errorcluster, "Alligator Queue Element 1 (+ 2)"=w510:T6[])  [unwired: 6 in]
    }
    frame "FLI Dataset:Square Gated IRF Characteristics Map" {
      # "Square Gated IRF Characteristics Map"
      n121 = call "Show Animated Busy Icon with Message and Abort Button.vi"("Already active? (F)"=w513, "Message"=w518, "Target VI reference"=w519) -> ("Error Out"=w522:errorcluster)  [unwired: 16 in]
      n122 = call "AlliGator Square Gated IRF Characteristics Map.vi"("error in (no error)"=w522, "AlliGator Internal Variables DVR"=w517) -> ("error out"=w521:errorcluster, "Message"=w515:string, "AlliGator Internal Variables DVR"=w516:refnum<data-value>)  [unwired: 7 in]
      n123 = call "Hide Animated Busy Icon with Message and Abort Button.vi"("Already active? (F)"=w513, "Target VI reference"=w519, "Error In"=w521) -> ("Error Out"=w514:errorcluster)  [unwired: 16 in]
    }
    frame "FLI Dataset:Tilted Logistic Square Gated IRF Characteristics Map" {
      # "Tilted Logistic Square Gated IRF Characteristics Map"
      n124 = Unbundle By Name(w528) -> ("Registered Events Ctrl Refnums.Decay Graph"=w533:refnum<vi>)
      n125 = call "AlliGator Get Square Gated IRF Analysis Cursors.vi"("XYGraph in"=w533) -> ("Error Out"=w537:errorcluster, "5 Cursors available?"=w534:bool, "Cursor Names Array"=w535:string[], "Cursor Positions Array"=w536:dbl[])  [unwired: 7 in]
      n126 = case shown="True" w534 {
        tunnel: w531 -> [_ w540]
        tunnel: w529 -> [_ w549]
        tunnel: w537 -> [w539 w543]
        tunnel: w536 -> [_ w548]
        tunnel: w535 -> [_ w547]
        tunnel: [w539 w542] -> w526
        tunnel: w532 -> [_ w546]
        tunnel: w527 -> [w538 w545]
        tunnel: [w538 w544] -> w524
        tunnel: [_ w541] -> w525
        frame False {
        }
        frame True {
          n127 = call "Show Animated Busy Icon with Message and Abort Button.vi"("Already active? (F)"=w540, "Message"=w549, "Target VI reference"=w546, "Error In"=w543) -> ("Error Out"=w551:errorcluster)  [unwired: 15 in]
          n128 = call "AlliGator Tilted Square Gated IRF Characteristics Map.vi"("error in (no error)"=w551, "Cursor Names Array"=w547, "Cursor Positions Array"=w548, "AlliGator Internal Variables DVR"=w545) -> ("error out"=w550:errorcluster, "Message"=w541:string, "AlliGator Internal Variables DVR"=w544:refnum<data-value>)  [unwired: 5 in]
          n129 = call "Hide Animated Busy Icon with Message and Abort Button.vi"("Already active? (F)"=w540, "Target VI reference"=w546, "Error In"=w550) -> ("Error Out"=w542:errorcluster)  [unwired: 16 in]
        }
      }
    }
    frame "FLI Dataset:Update Decay Statistics Graph" {
      # "Update Decay Statistics Graph"
      n130 = call "AlliGator IV Decays Max & Min.vi"("Set (T)/Get (F)"=FALSE, "AlliGator IV DVR in"=w557) -> ("Error Out"=w561:errorcluster, "[Decays Min Value]"=w562:sgl[], "[Decays Max Value]"=w563:sgl[], "AlliGator IV DVR out"=w556:refnum<data-value>)  [unwired: 6 in]
      n131 = Unbundle By Name(w558) -> ("Registered Events Ctrl Refnums.Decay Statistics Graph"=w566:refnum<vi>, "Other AlliGator Ctrl Refnums.Decay Statistics Bin"=w565:refnum<vi>)
      n132 = property class="DigNum (strict)"(reference=w565) -> ("Value"=w564:i32)  [unwired: 1 in, 2 out]
      n133 = call "Show Animated Busy Icon with Message.vi"("Already active? (F)"=w552, "Message"=w553, "Error In"=w561, "Target VI Refnum"=w559) -> ("Error Out"=w567:errorcluster)  [unwired: 7 in]
      n134 = call "AlliGator Recompute Decay Statistics Histograms.vi"("Decay Statistics Graph"=w566, "Error In"=w567, "Decay Statistics Bin"=w564, "Decays Min Values"=w562, "Decays Max Values"=w563) -> ("Error Out"=w568:errorcluster)  [unwired: 6 in]
      n135 = call "Hide Animated Busy Icon with Message.vi"("Already active? (F)"=w552, "Error In"=w568, "Target VI reference"=w559) -> ("Error Out"=w554:errorcluster)  [unwired: 8 in]
    }
    frame "FLI Dataset:Phasor Calibration Maps (# Gates Series) Script" {
      # "FLI Dataset:Phasor Calibration Maps (# Gates Series) Script"
      n136 = call "AlliGator Phasor Calibration Map Series Dialog.vi"("error in (no error)"=w573) -> ("File Name (# Steps will be added)"=w584:string, "Destination Folder"=w583:path, "Gate Step Series"=w582:string, "Phasor Calibration Dataset Path"=w581:path, "OK"=w579:bool, "error out"=w580:errorcluster)  [unwired: 13 in]
      n137 = Unbundle By Name(w572) -> ("Registered Events Ctrl Refnums.Phasor Graph"=w578:refnum<vi>)
      n138 = case shown="True" w579 {
        tunnel: w577 -> [w587 w601]
        tunnel: [w587 w600] -> w576
        tunnel: w584 -> [_ w599]
        tunnel: w583 -> [_ w598]
        tunnel: w582 -> [_ w597]
        tunnel: w581 -> [_ w596]
        tunnel: w580 -> [w586 w595]
        tunnel: w578 -> [_ w594]
        tunnel: w570 -> [_ w588]
        tunnel: w569 -> [_ w593]
        tunnel: [w586 w592] -> w574
        tunnel: w571 -> [_ w590]
        tunnel: [_ w589] -> w575
        frame False {
        }
        frame True {
          n139 = call "AlliGator Phasor Calibration Maps (# Gates Series) Script.vi"("Alligator Queue Elements in"=w601, "Phasor Graph refnum"=w594, "File Name (# Steps will be added)"=w599, "Destination Folder"=w598, "Gate Step Series"=w597, "Error In"=w595, "Phasor Calibration Dataset Path"=w596) -> ("Alligator Queue Elements out"=w600:T6[], "Message"=w589:string, "Error Out"=w591:errorcluster)  [unwired: 6 in]
          n140 = call "Show Animated Busy Icon with Message and Abort Button.vi"("Already active? (F)"=w588, "Message"=w593, "Target VI reference"=w590, "Error In"=w591) -> ("Error Out"=w592:errorcluster)  [unwired: 15 in]
        }
      }
    }
    frame "FLI Dataset:Calibrated Phasor Map Series" {
      # "FLI Dataset:Calibrated Phasor Map Series"
      n141 = Unbundle By Name(w610) -> ("Registered Events Ctrl Refnums.Phasor Graph"=w612:refnum<vi>)
      n142 = call "AlliGator Calibrated Phasor Map Series Dialog.vi"("error in (no error)"=w608) -> ("OK"=w613:bool, "Calibration Map/Gate Step List"=w617:T51[], "Destination Folder"=w616:path, "File Suffix (# Steps will be added)"=w615:string, "Save Phasor Plot"=w614:bool, "error out"=w618:errorcluster)  [unwired: 13 in]
      n143 = case shown="True" w613 {
        tunnel: w611 -> [w622 w634]
        tunnel: [w622 w633] -> w607
        tunnel: w618 -> [w621 w631]
        tunnel: w612 -> [_ w632]
        tunnel: w604 -> [w620 w623]
        tunnel: w602 -> [_ w638]
        tunnel: [w621 w637] -> w609
        tunnel: [w620 w635] -> w603
        tunnel: w617 -> [_ w630]
        tunnel: w616 -> [_ w629]
        tunnel: w615 -> [_ w628]
        tunnel: w614 -> [_ w627]
        tunnel: w605 -> [_ w625]
        tunnel: [_ w624] -> w606
        frame False {
        }
        frame True {
          n144 = call "AlliGator Calibrated Phasor Maps Series Script.vi"("Alligator Queue Elements in"=w634, "Calibration Map/Gate Step List"=w630, "Destination Folder"=w629, "File Suffix (# Steps will be added)"=w628, "Save Phasor Plot"=w627, "Error In"=w631, "Phasor Graph refnum"=w632) -> ("Alligator Queue Elements out"=w633:T6[], "Message"=w624:string, "Error Out"=w626:errorcluster)  [unwired: 10 in]
          n145 = call "Show Animated Busy Icon with Message and Abort Button.vi"("Already active? (F)"=w623, "Message"=w638, "Target VI reference"=w625, "Error In"=w626) -> ("Error Out"=w637:errorcluster)  [unwired: 15 in]
          n146 = Unbundle By Name(w637) -> ("status"=w636:bool)
          n147 = Not(x=w636) -> (.not. x?=w635:bool)
        }
      }
    }
  }
  "AlliGator IV DVR out" <- w17
  "error out" <- w6
  "Script out" <- w10
  "Alligator Queue Elements" <- w9
  n148 = call "Get Current Message Text Format.vi"("Text Format"=w1) -> ("Message Formatting"=w2:T2)  [unwired: 8 in, 1 out]
  n149 = call "AlliGator Package Notebook Messages.vi"("Message Formatting"=w2, "Message"=w4, "AlliGator Q Event in"="AlliGator Q Event in") -> ("[Notebook Message]"=→"[Notebook Message]":T1[])  [unwired: 8 in]
